vi "doComms.vi"(1 "Initialization":T1={"connID"=refnum, "client"="", "OpenFP"=TRUE, "useAuthentication"=FALSE, "DSN"="", "Package Size"=1, "Sending Rate (ms)"=100, "error"={"status"=FALSE, "code"=0, "source"=""}} {"Sending Rate (ms)" min=1 max=1000 step=1; "Package Size" min=1 max=1000 step=1}) -> ()   [LabVIEW 2010]
panel:
  out "starttime":string
  out "endtime":string
  out "Indicators formated":cluster{"name":string, "type desc":i16[]}[](array[cluster])
  out "Controls formated":cluster{"name":string, "type desc":i16[]}[](array[cluster])
  out "output Indicators":cluster{"name":string, "type desc":i16[]}[](array[cluster])
  out "output Controls":cluster{"name":string, "type desc":i16[]}[](array[cluster])
  out "vi reference":refnum<vi>
  out "Execution: State VI":T2(ring)
  out "Application":string
  out "Application absolute path":path
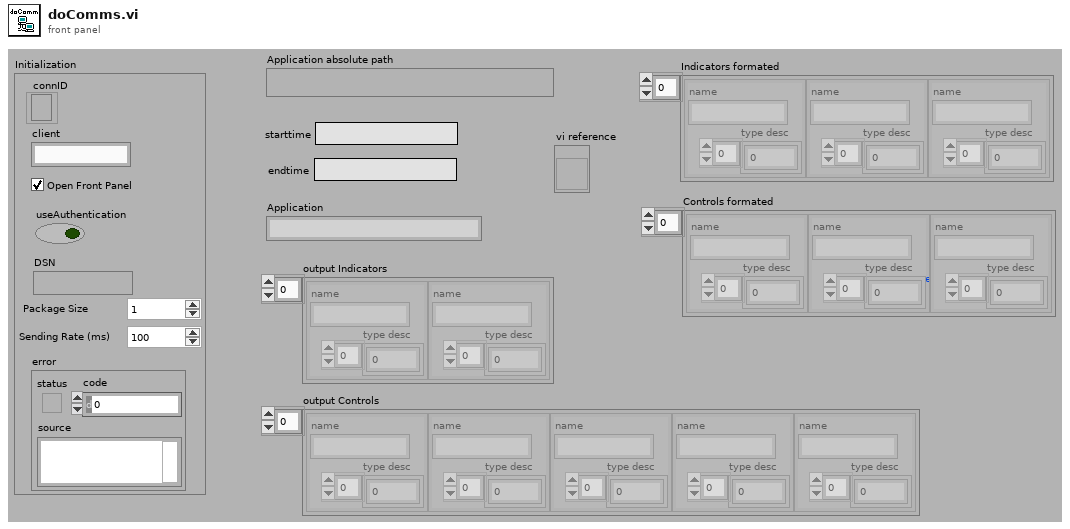
[diagram p1: front panel]
types:
  T1 = cluster{"connID":refnum<k5>, "client":string, "OpenFP":bool, "useAuthentication":bool, "DSN":string, "Package Size":u32, "Sending Rate (ms)":u32, "error":errorcluster}
  T2 = enum16{"Bad", "Idle", "Run top level", "Running"}
  T3 = enum32{"Bad", "Idle", "Run top level", "Running"}
  T4 = enum16{"open", "replace", "create", "open or create", "replace or create", "replace or create with confirmation"}
  T5 = typedef "imagedata.ctl" = cluster{"image type":i32, "image depth":i32, "image":u8[], "mask":u8[], "colors":u32[], "Rectangle":cluster{"left":i16, "top":i16, "right":i16, "bottom":i16}}
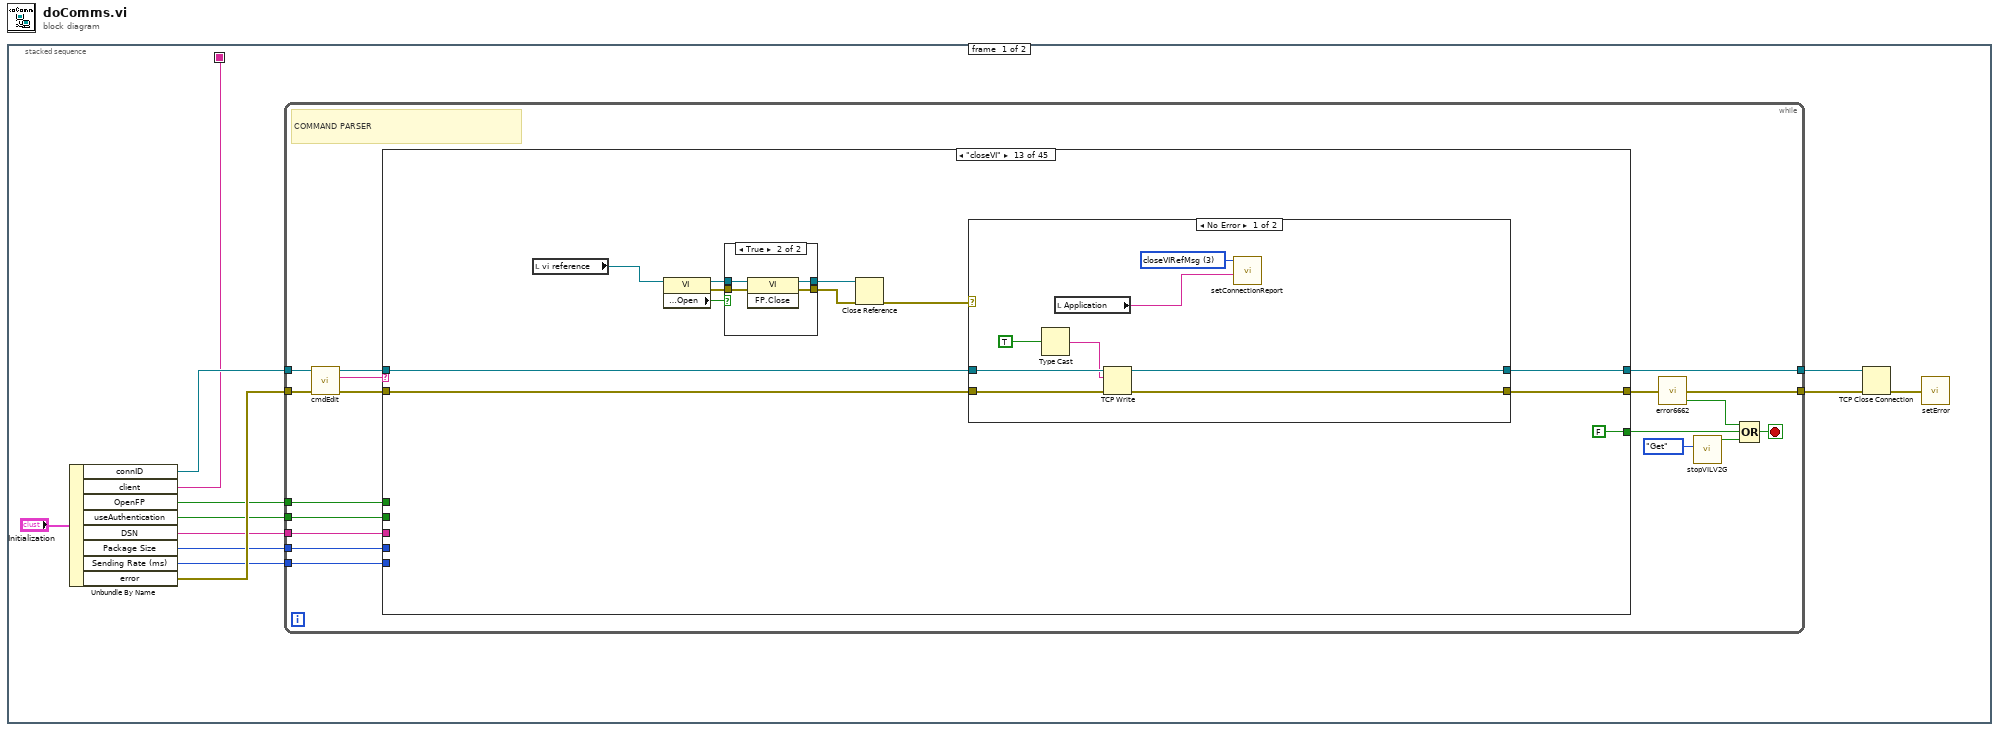
[diagram p0: block diagram]
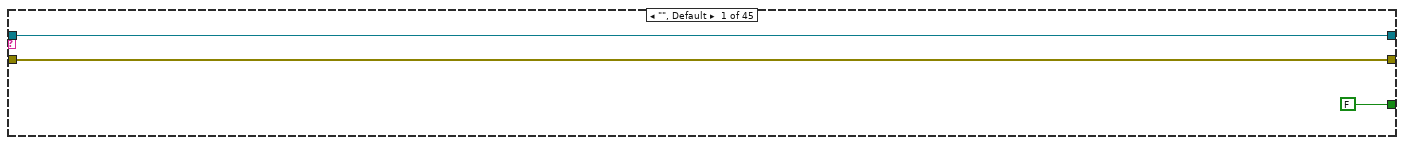
[diagram p2: hidden frame]
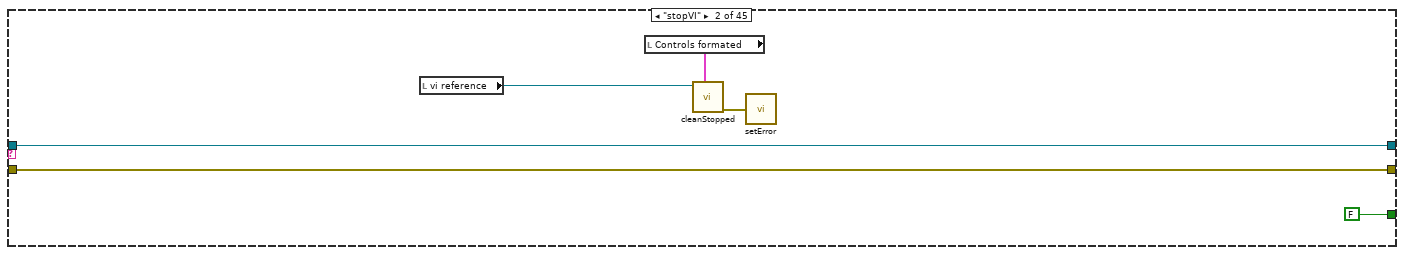
[diagram p3: hidden frame]
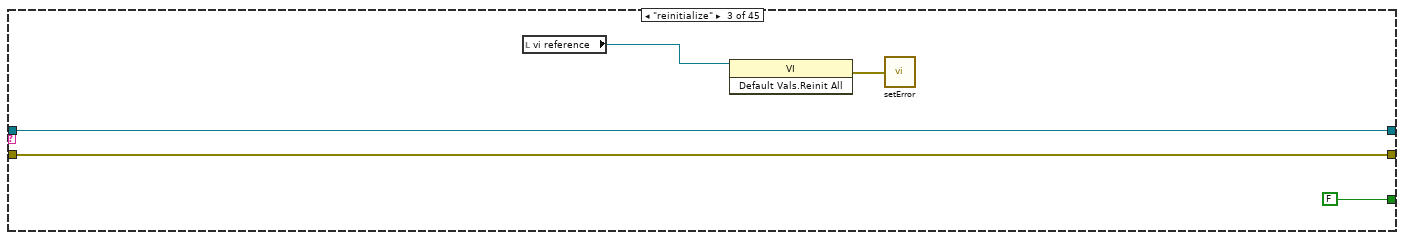
[diagram p4: hidden frame]
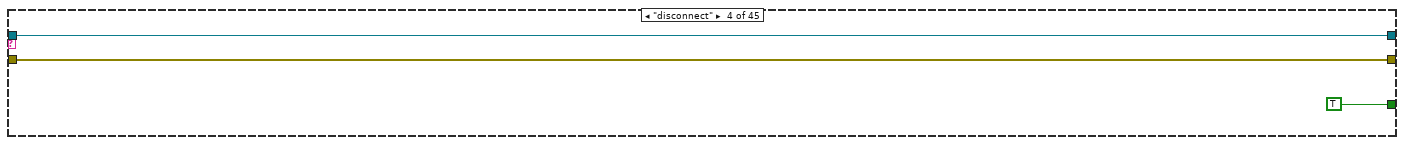
[diagram p5: hidden frame]
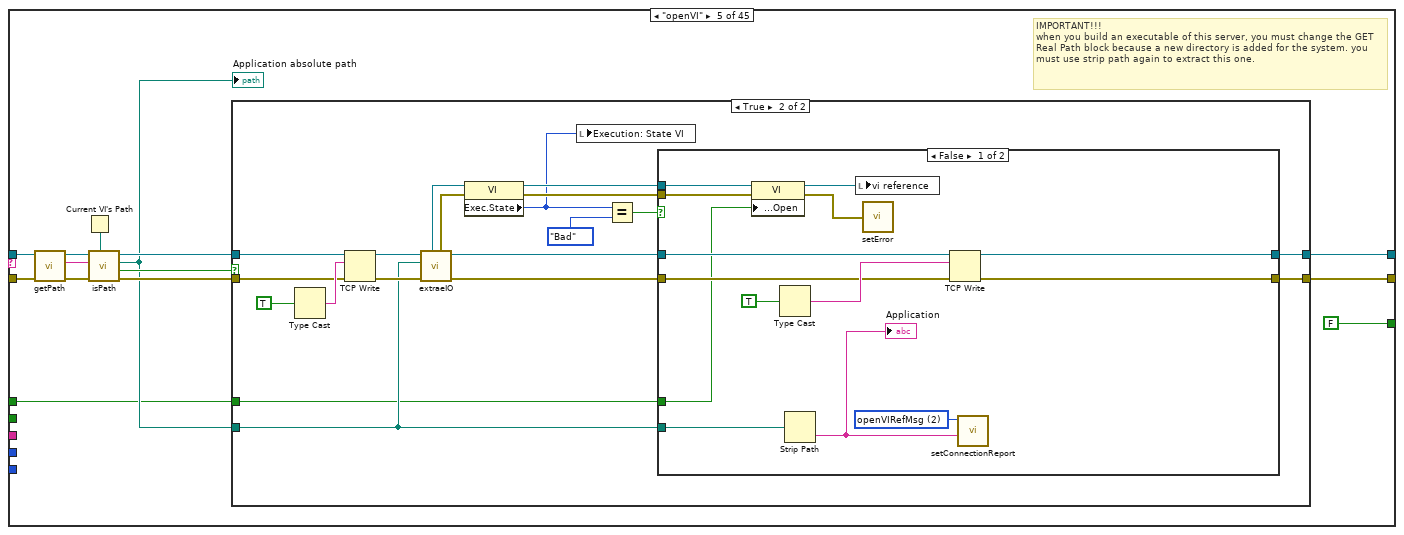
[diagram p6: hidden frame]
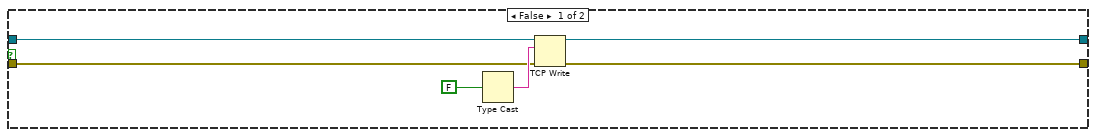
[diagram p7: hidden frame]
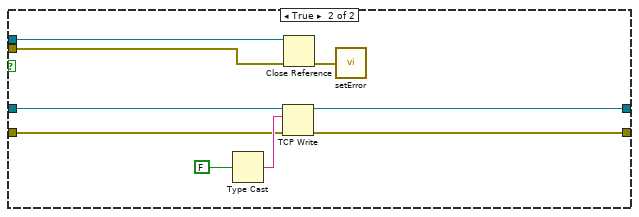
[diagram p8: hidden frame]
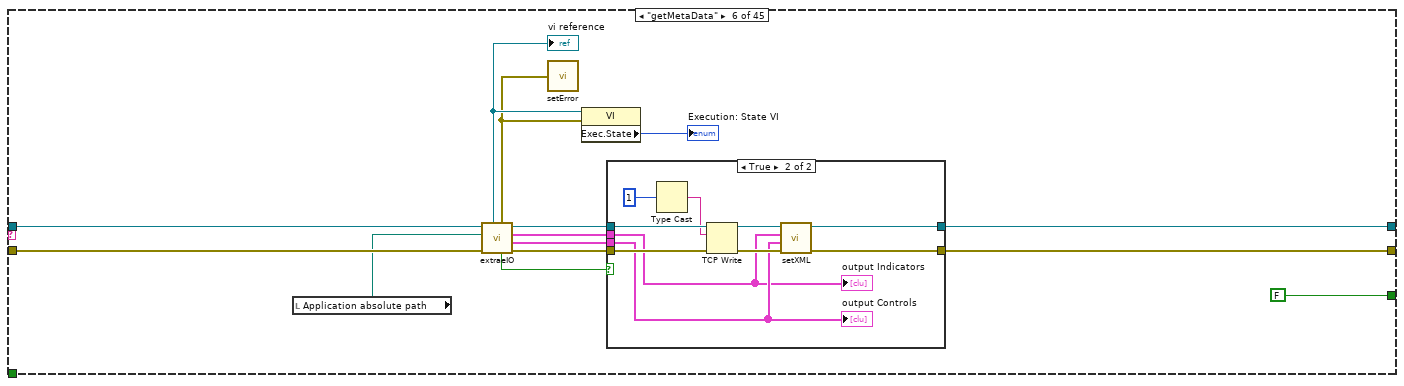
[diagram p9: hidden frame]
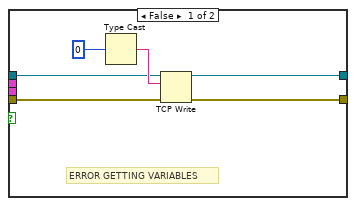
[diagram p10: hidden frame]
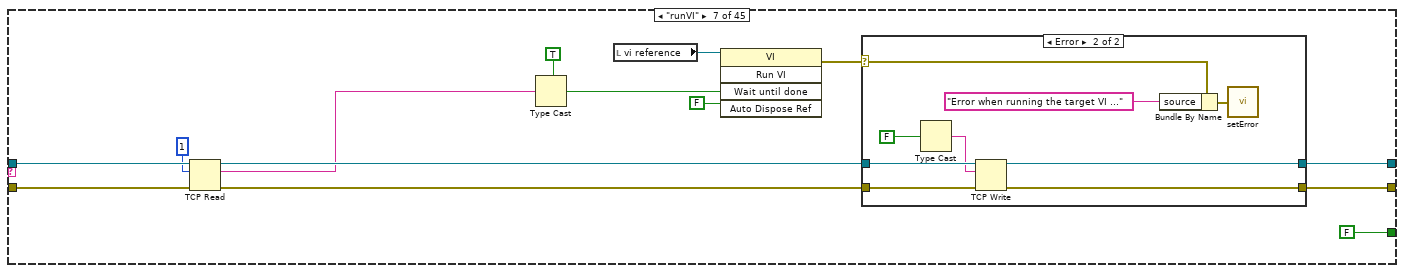
[diagram p11: hidden frame]
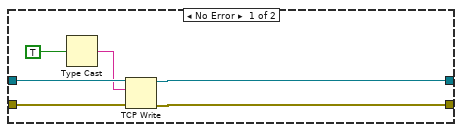
[diagram p12: hidden frame]
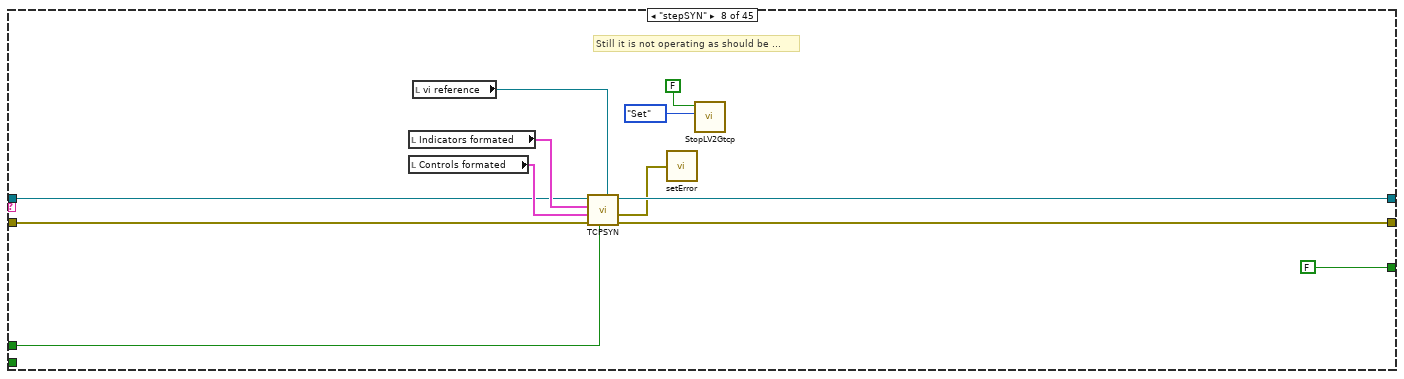
[diagram p13: hidden frame]
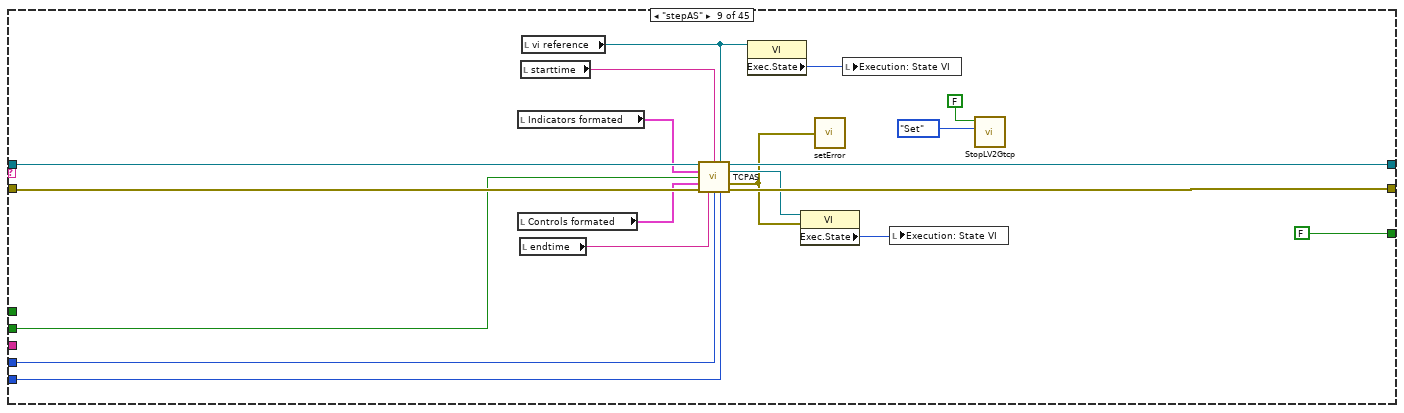
[diagram p14: hidden frame]
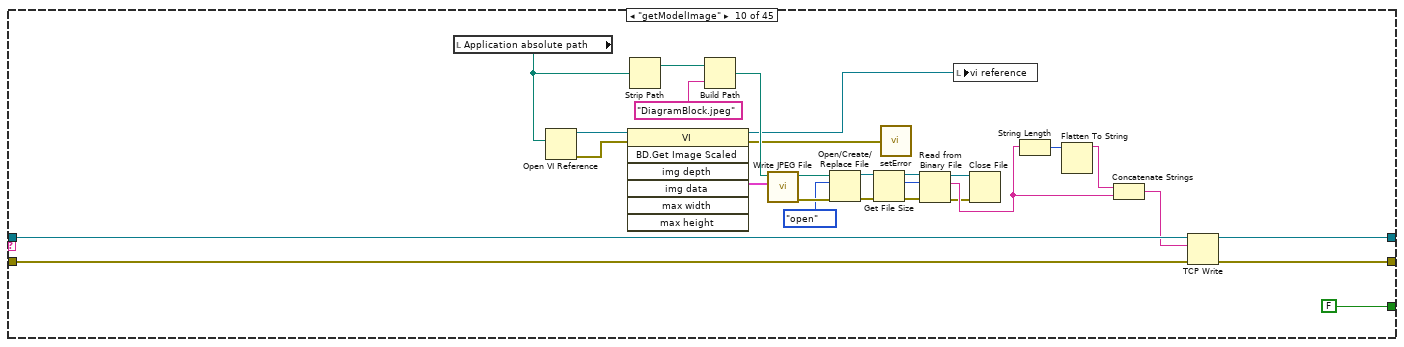
[diagram p15: hidden frame]
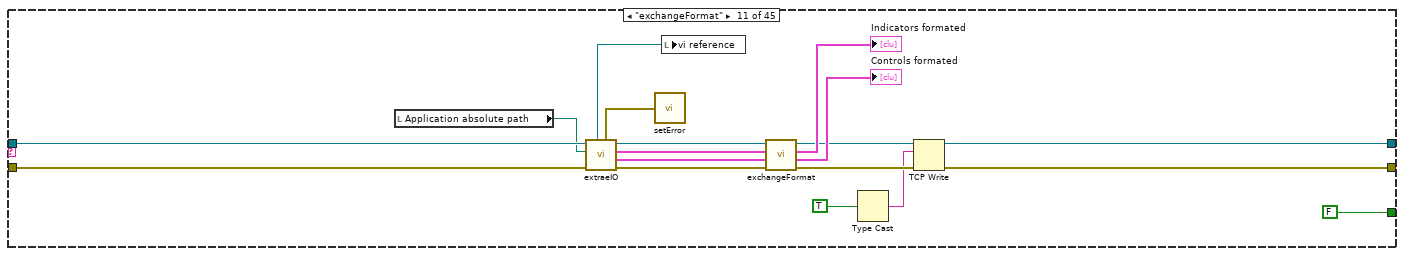
[diagram p16: hidden frame]
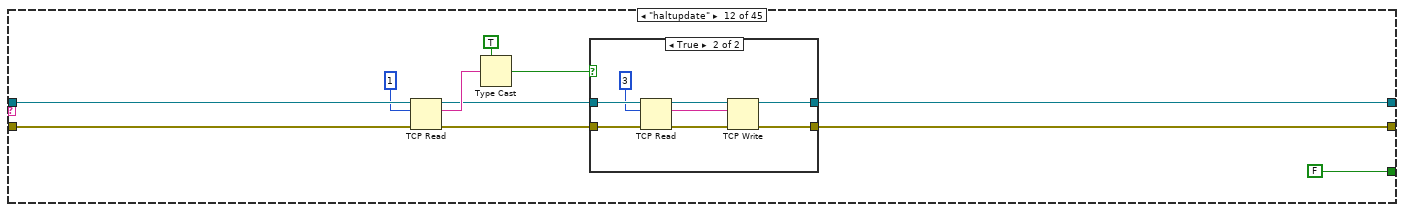
[diagram p17: hidden frame]
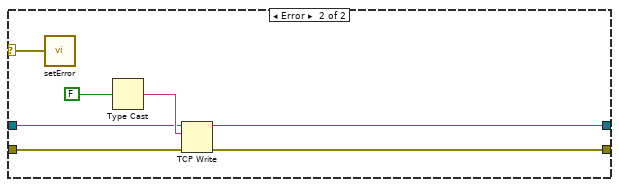
[diagram p19: hidden frame]
diagram:
  n1 = stacked-sequence {
    seq-local: [w1 _] -> [_ w1190]
    frame #0 {
      n2 = Unbundle By Name("Initialization") -> ("connID"=w8:refnum<k5>, "client"=w1:string, "OpenFP"=w5:bool, "useAuthentication"=w6:bool, "DSN"=w2:string, "Package Size"=w4:u32, "Sending Rate (ms)"=w3:u32, "error"=w7:errorcluster)
      n3 = while {
        tunnel: w8 -> [w29]
        tunnel: w7 -> [w28]
        tunnel: [w23] -> w12
        tunnel: [w30] -> w11
        tunnel: w6 -> [w17]
        tunnel: w5 -> [w16]
        tunnel: w4 -> [w15]
        tunnel: w3 -> [w14]
        tunnel: w2 -> [w13]
        stop <- w22 stop-if-true
        # "COMMAND PARSER"
        n4 = call "cmdEdit.vi"("error in (no error)"=w28, "connection ID"=w29) -> ("error out"=w26:errorcluster, "Command"=w25:string, "connection ID out"=w27:refnum<k5>)  [unwired: 7 out]
        n5 = case shown="\"closeVI\"" w25 {
          tunnel: w27 -> [w33 w38 w43 w47 w57 w117 w152 w177 w196 w221 w245 w256 w271 w314 w351 w359 w384 w407 w430 w461 w485 w515 w551 w590 w623 w661 w700 w739 w780 w827 w871 w890 w912 w934 w955 w978 w1000 w1022 w1044 w1065 w1088 w1110 w1132 w1150 w1173]
          tunnel: w26 -> [w32 w37 w42 w46 w56 w116 w151 w176 w195 w220 w244 w255 w270 w313 w350 w358 w383 w406 w429 w460 w484 w516 w550 w589 w622 w660 w699 w738 w779 w826 w870 w889 w911 w933 w954 w977 w999 w1021 w1043 w1064 w1087 w1109 w1131 w1149 w1172]
          tunnel: [w32 w37 w42 w46 w51 w122 w148 w175 w192 w225 w232 w246 w267 w303 w350 w357 w382 w404 w428 w459 w483 w517 w549 w581 w625 w658 w697 w737 w773 w825 w865 w888 w910 w932 w953 w976 w998 w1020 w1042 w1062 w1085 w1108 w1130 w1152 w1171] -> w24
          tunnel: [w33 w38 w43 w47 w52 w123 w149 w174 w191 w226 w231 w247 w268 w304 w351 w356 w381 w405 w427 w458 w482 w518 w552 w582 w624 w659 w698 w736 w774 w824 w863 w887 w909 w931 w952 w975 w997 w1019 w1041 w1063 w1086 w1107 w1129 w1153 w1170] -> w30
          tunnel: [FALSE FALSE FALSE TRUE FALSE FALSE FALSE FALSE FALSE FALSE FALSE FALSE FALSE FALSE FALSE FALSE FALSE FALSE FALSE FALSE FALSE FALSE FALSE FALSE FALSE FALSE FALSE FALSE FALSE FALSE FALSE FALSE FALSE FALSE FALSE FALSE FALSE FALSE FALSE FALSE FALSE FALSE FALSE FALSE FALSE] -> w20
          tunnel: w17 -> [_ _ _ _ _ _ _ _ w188 _ _ _ _ _ _ _ _ _ _ _ _ _ _ _ _ _ _ _ _ _ _ _ _ _ _ _ _ _ _ _ _ _ _ _ _]
          tunnel: w16 -> [_ _ _ _ w48 _ _ w169 _ _ _ _ _ _ _ _ _ _ _ _ _ _ _ _ _ _ _ _ _ _ _ _ _ _ _ _ _ _ _ _ _ _ _ _ _]
          tunnel: w15 -> [_ _ _ _ _ _ _ _ w182 _ _ _ _ _ _ _ _ _ _ _ _ _ _ _ _ _ _ _ _ _ _ _ _ _ _ _ _ _ _ _ _ _ _ _ _]
          tunnel: w14 -> [_ _ _ _ _ _ _ _ w181 _ _ _ _ _ _ _ _ _ _ _ _ _ _ _ _ _ _ _ _ _ _ _ _ _ _ _ _ _ _ _ _ _ _ _ _]
          tunnel: w13 -> [_ _ _ _ _ _ _ _ _ _ _ _ _ w300 _ _ _ _ _ _ _ _ _ _ _ _ _ _ _ _ _ _ _ _ _ _ _ _ _ _ _ _ _ _ _]
          frame "", Default {
          }
          frame "stopVI" {
            n6 = local read "vi reference"() -> (w36:refnum<vi>)
            n7 = local read "Controls formated"() -> (w35:cluster{"name":string, "type desc":i16[]}[])
            n8 = call "cleanStopped.vi"("input Controls"=w35, "vi reference in"=w36) -> ("error out"=w34:errorcluster)  [unwired: 1 in, 8 out]
            n9 = call "setError.vi"("error"=w34) -> ()  [unwired: 1 out]
          }
          frame "reinitialize" {
            n10 = local read "vi reference"() -> (w41:refnum<vi>)
            n11 = invoke class="VI" method="Default Vals.Reinit All"(reference=w41) -> (error out=w40:errorcluster)  [unwired: 2 in, 2 out]
            n12 = call "setError.vi"("error"=w40) -> ()  [unwired: 1 out]
          }
          frame "disconnect" {
          }
          frame "openVI" {
            # "IMPORTANT!!!\nwhen you build an executable of this server, you must change the GET Real Path block because a new directory is added for the system. you must use strip path again to extract this one."
            n13 = call "getPath.vi"("error in TCP"=w56, "connection ID in"=w57) -> ("error out TCP"=w58:errorcluster, "name vi"=w61:string, "connection ID out"=w59:refnum<k5>)  [unwired: 7 out]
            n14 = Current VI's Path() -> (path=w60:path)
            n15 = call "isPath.vi"("path Current VI"=w60, "error in TCP"=w58, "string Path in"=w61, "connection ID in"=w59) -> ("error out TCP"=w54:errorcluster, "Path is Ok?"=w55:bool, "absolute path"=w49:path, "connection ID out"=w53:refnum<k5>)  [unwired: 4 out]
            "Application absolute path" <- w49
            n16 = case shown="True" w55 {
              tunnel: w54 -> [w64 w83]
              tunnel: w53 -> [w65 w84]
              tunnel: [w62 w71] -> w52
              tunnel: [w63 w72] -> w51
              tunnel: w49 -> [_ w70]
              tunnel: w48 -> [_ w68]
              frame False {
                n17 = Type Cast(x=FALSE) -> (*(type *) &x=w67:string)  [unwired: 1 out]
                n18 = TCP Write(connection ID=w65, data in=w67, error in (no error)=w64) -> (connection ID out=w62:refnum<k5>, error out=w63:errorcluster)  [unwired: 2 out]
              }
              frame True {
                n19 = Type Cast(x=TRUE) -> (*(type *) &x=w86:string)  [unwired: 1 out]
                n20 = TCP Write(connection ID=w84, data in=w86, error in (no error)=w83) -> (connection ID out=w82:refnum<k5>, error out=w81:errorcluster)  [unwired: 2 out]
                n21 = call "extraeIO.vi"("error in TCP"=w81, "path"=w70, "connection IDin"=w82) -> ("error out TCP"=w73:errorcluster, "connection ID out"=w74:refnum<k5>, "error out"=w79:errorcluster, "vi reference"=w80:refnum<vi>)  [unwired: 5 out]
                n22 = property class="VI"(reference=w80, error in=w79) -> (reference out=w76:refnum<vi>, error out=w75:errorcluster, "Exec.State"=w69:T3)
                n23 = local write "Execution: State VI"(w69) -> ()
                n24 = Equal?(x=w69, y=T3."Bad") -> (x = y?=w78:bool)
                n25 = case shown="False" w78 {
                  tunnel: w76 -> [w92 w106]
                  tunnel: w75 -> [w91 w107]
                  tunnel: w74 -> [w96 w105]
                  tunnel: w73 -> [w95 w104]
                  tunnel: [w94 w103] -> w72
                  tunnel: [w93 w102] -> w71
                  tunnel: w70 -> [w97 _]
                  tunnel: w68 -> [w87 _]
                  frame False {
                    w88 = u16 2 items=["connectedMsg", "disconnectedMsg", "openVIRefMsg", "closeVIRefMsg"] ("Type of Message")
                    n26 = property class="VI"(reference=w92, error in=w91, "Front Panel.Open"=w87) -> (reference out=w98:refnum<vi>, error out=w90:errorcluster)
                    n27 = Type Cast(x=TRUE) -> (*(type *) &x=w100:string)  [unwired: 1 out]
                    n28 = Strip Path(path=w97) -> (name=w89:string)  [unwired: 1 out]
                    "Application" <- w89
                    n29 = local write "vi reference"(w98) -> ()
                    n30 = call "setError.vi"("error"=w90) -> ()  [unwired: 1 out]
                    n31 = TCP Write(connection ID=w96, data in=w100, error in (no error)=w95) -> (connection ID out=w93:refnum<k5>, error out=w94:errorcluster)  [unwired: 2 out]
                    n32 = call "setConnectionReport.vi"("string"=w89, "Type of Message"=w88) -> ()  [unwired: 10 in]
                  }
                  frame True {
                    n33 = Type Cast(x=FALSE) -> (*(type *) &x=w109:string)  [unwired: 1 out]
                    n34 = TCP Write(connection ID=w105, data in=w109, error in (no error)=w104) -> (connection ID out=w102:refnum<k5>, error out=w103:errorcluster)  [unwired: 2 out]
                    n35 = Close Reference(reference=w106, error in (no error)=w107) -> (error out=w101:errorcluster)
                    n36 = call "setError.vi"("error"=w101) -> ()  [unwired: 1 out]
                  }
                }
              }
            }
          }
          frame "getMetaData" {
            n37 = local read "Application absolute path"() -> (w115:path)
            n38 = call "extraeIO.vi"("error in TCP"=w116, "path"=w115, "connection IDin"=w117) -> ("error out TCP"=w119:errorcluster, "output Controls"=w113:cluster{"name":string, "type desc":i16[]}[], "output Indicators"=w120:cluster{"name":string, "type desc":i16[]}[], "connection ID out"=w118:refnum<k5>, "it is ok?"=w114:bool, "error out"=w110:errorcluster, "vi reference"=w112:refnum<vi>)  [unwired: 2 out]
            "vi reference" <- w112
            n39 = call "setError.vi"("error"=w110) -> ()  [unwired: 1 out]
            n40 = property class="VI"(reference=w112, error in=w110) -> ("Exec.State"=→"Execution: State VI":T3)  [unwired: 2 out]
            n41 = case shown="True" w114 {
              tunnel: w119 -> [w129 w136]
              tunnel: w120 -> [_ w130]
              tunnel: w113 -> [_ w131]
              tunnel: [w127 w139] -> w123
              tunnel: [w128 w138] -> w122
              tunnel: w118 -> [w124 w137]
              frame False {
                # "ERROR GETTING VARIABLES"
                n42 = Type Cast(x=0) -> (*(type *) &x=w126:string)  [unwired: 1 out]
                n43 = TCP Write(connection ID=w124, data in=w126, error in (no error)=w129) -> (connection ID out=w127:refnum<k5>, error out=w128:errorcluster)  [unwired: 2 out]
              }
              frame True {
                n44 = Type Cast(x=1) -> (*(type *) &x=w132:string)  [unwired: 1 out]
                n45 = TCP Write(connection ID=w137, data in=w132, error in (no error)=w136) -> (connection ID out=w134:refnum<k5>, error out=w135:errorcluster)  [unwired: 2 out]
                n46 = call "setXML.vi"("error in"=w135, "Controls filtered"=w131, "Indicators filtered"=w130, "connection ID in"=w134) -> ("error out"=w138:errorcluster, "connection ID out"=w139:refnum<k5>)  [unwired: 6 out]
                "output Indicators" <- w130
                "output Controls" <- w131
              }
            }
          }
          frame "runVI" {
            n47 = TCP Read(connection ID=w152, bytes to read=1, error in (no error)=w151) -> (connection ID out=w147:refnum<k5>, data out=w142:string, error out=w146:errorcluster)  [unwired: 2 out]
            n48 = Type Cast(type=TRUE, x=w142) -> (*(type *) &x=w145:bool)
            n49 = local read "vi reference"() -> (w141:refnum<vi>)
            n50 = invoke class="VI" method="Run VI"(reference=w141, "Wait until done"=w145, "Auto Dispose Ref"=FALSE ("Auto Dispose Reference")) -> (error out=w150:errorcluster)  [unwired: 2 in, 4 out]
            n51 = case shown="Error" w150 {
              selector: w150 -> [_ w161]
              tunnel: w147 -> [w159 w168]
              tunnel: w146 -> [w158 w167]
              tunnel: [w157 w166] -> w149
              tunnel: [w156 w165] -> w148
              frame No Error {
                n52 = Type Cast(x=TRUE) -> (*(type *) &x=w154:string)  [unwired: 1 out]
                n53 = TCP Write(connection ID=w159, data in=w154, error in (no error)=w158) -> (connection ID out=w157:refnum<k5>, error out=w156:errorcluster)  [unwired: 2 out]
              }
              frame Error {
                n54 = Type Cast(x=FALSE) -> (*(type *) &x=w163:string)  [unwired: 1 out]
                n55 = TCP Write(connection ID=w168, data in=w163, error in (no error)=w167) -> (connection ID out=w166:refnum<k5>, error out=w165:errorcluster)  [unwired: 2 out]
                n56 = Bundle By Name(cluster=w161, "source"="Error when running the target VI ...") -> (w160:errorcluster)
                n57 = call "setError.vi"("error"=w160) -> ()  [unwired: 1 out]
              }
            }
          }
          frame "stepSYN" {
            # "Still it is not operating as should be ..."
            n58 = local read "Indicators formated"() -> (w180:cluster{"name":string, "type desc":i16[]}[])
            n59 = local read "Controls formated"() -> (w179:cluster{"name":string, "type desc":i16[]}[])
            n60 = local read "vi reference"() -> (w178:refnum<vi>)
            n61 = call "TCPSYN.vi"("vi reference"=w178, "Front Panel Window:Open"=w169, "error in TCP"=w176, "input Controls"=w179, "input Indicators"=w180, "connection ID in"=w177) -> ("error TCP out"=w175:errorcluster, "error out"=w170:errorcluster, "connection ID out"=w174:refnum<k5>)  [unwired: 1 in, 2 out]
            n62 = call "setError.vi"("error"=w170) -> ()  [unwired: 1 out]
            n63 = call "StopLV2Gtcp.vi"("Mode"=enum16{"Init", "Get", "Set"}."Set", "Stop IN"=FALSE) -> ()  [unwired: 10 out]
          }
          frame "stepAS" {
            n64 = local read "Indicators formated"() -> (w194:cluster{"name":string, "type desc":i16[]}[])
            n65 = local read "Controls formated"() -> (w193:cluster{"name":string, "type desc":i16[]}[])
            n66 = local read "endtime"() -> (w189:string)
            n67 = local read "starttime"() -> (w190:string)
            n68 = local read "vi reference"() -> (w187:refnum<vi>)
            n69 = call "TCPAS.vi"("connection ID in"=w196, "starttime"=w190, "vi reference"=w187, "input Indicators"=w194, "rejectbyendtime"=w188, "input Controls"=w193, "error in TCP"=w195, "endtime"=w189, "packageSize"=w182, "Sent rate (ms)"=w181) -> ("connection ID out"=w191:refnum<k5>, "vi reference"=w185:refnum<vi>, "error out"=w183:errorcluster, "error TCP out"=w192:errorcluster)  [unwired: 1 in, 1 out]
            n70 = property class="VI"(reference=w187) -> ("Exec.State"=w186:T3)  [unwired: 1 in, 2 out]
            n71 = property class="VI"(reference=w185, error in=w183) -> ("Exec.State"=w184:T3)  [unwired: 2 out]
            n72 = call "setError.vi"("error"=w183) -> ()  [unwired: 1 out]
            n73 = local write "Execution: State VI"(w186) -> ()
            n74 = local write "Execution: State VI"(w184) -> ()
            n75 = call "StopLV2Gtcp.vi"("Mode"=enum16{"Init", "Get", "Set"}."Set", "Stop IN"=FALSE) -> ()  [unwired: 10 out]
          }
          frame "getModelImage" {
            n76 = local read "Application absolute path"() -> (w219:path)
            n77 = Open VI Reference(vi path=w219) -> (vi reference=w218:refnum<vi>, error out=w217:errorcluster)  [unwired: 1 in, 4 out]
            n78 = invoke class="VI" method="BD.Get Image Scaled"(reference=w218, error in=w217) -> (reference out=w216:refnum<vi>, error out=w200:errorcluster, "img data"=w215:T5)  [unwired: 5 in, 4 out]
            n79 = Strip Path(path=w219) -> (stripped path=w224:path)  [unwired: 1 out]
            n80 = Build Path(base path=w224, name or relative path="DiagramBlock.jpeg") -> (appended path=w222:path)
            n81 = call <vilib>:"Write JPEG File.vi"("image data"=w215, "path to JPEG file"=w222) -> ("error out"=w208:errorcluster, "path"=w209:path)  [unwired: 1 in, 7 out]
            n82 = Open/Create/Replace File(file path (use dialog)=w209, error in=w208, operation (0:open)=T4."open") -> (refnum out=w210:refnum<file>, error out=w211:errorcluster)  [unwired: 4 out]
            n83 = Get File Size(file=w210, error in=w211) -> (refnum out=w206:refnum<file>, size (in bytes)=w205:i64, 0:w204:errorcluster)
            n84 = call "setError.vi"("error"=w200) -> ()  [unwired: 1 out]
            n85 = Read from Binary File(8:w204, 10:w205, 11:w206) -> (0:w202:errorcluster, 2:w214:string, 3:w203:refnum<file>)  [unwired: 4 out]
            n86 = local write "vi reference"(w216) -> ()
            n87 = Close File(refnum=w203, error in=w202) -> ()  [unwired: 2 out]
            n88 = String Length(string=w214) -> (length=w201:i32)
            n89 = Flatten To String(anything=w201) -> (data string=w213:string)  [unwired: 1 in, 4 out]
            n90 = Concatenate Strings(w213, w214) -> (w212:string)
            n91 = TCP Write(connection ID=w221, data in=w212, error in (no error)=w220) -> (connection ID out=w226:refnum<k5>, error out=w225:errorcluster)  [unwired: 2 out]
          }
          frame "exchangeFormat" {
            n92 = local read "Application absolute path"() -> (w243:path)
            n93 = call "extraeIO.vi"("error in TCP"=w244, "path"=w243, "connection IDin"=w245) -> ("error out TCP"=w239:errorcluster, "output Controls"=w237:cluster{"name":string, "type desc":i16[]}[], "output Indicators"=w238:cluster{"name":string, "type desc":i16[]}[], "connection ID out"=w240:refnum<k5>, "error out"=w228:errorcluster, "vi reference"=w241:refnum<vi>)  [unwired: 3 out]
            n94 = call "setError.vi"("error"=w228) -> ()  [unwired: 1 out]
            n95 = local write "vi reference"(w241) -> ()
            n96 = call "exchangeFormat.vi"("error in TCP"=w239, "input Controls"=w237, "input Indicators"=w238, "connection ID in"=w240) -> ("error out TCP"=w233:errorcluster, "output Controls"=→"Controls formated":cluster{"name":string, "type desc":i16[]}[], "output Indicators"=→"Indicators formated":cluster{"name":string, "type desc":i16[]}[], "connection ID out"=w234:refnum<k5>)  [unwired: 4 out]
            n97 = Type Cast(x=TRUE) -> (*(type *) &x=w230:string)  [unwired: 1 out]
            n98 = TCP Write(connection ID=w234, data in=w230, error in (no error)=w233) -> (connection ID out=w231:refnum<k5>, error out=w232:errorcluster)  [unwired: 2 out]
          }
          frame "haltupdate" {
            n99 = TCP Read(connection ID=w256, bytes to read=1, error in (no error)=w255) -> (connection ID out=w249:refnum<k5>, data out=w253:string, error out=w248:errorcluster)  [unwired: 2 out]
            n100 = Type Cast(type=TRUE, x=w253) -> (*(type *) &x=w251:bool)
            n101 = case shown="True" w251 {
              tunnel: w249 -> [w258 w266]
              tunnel: w248 -> [w257 w265]
              tunnel: [w258 w260] -> w247
              tunnel: [w257 w259] -> w246
              frame False {
              }
              frame True {
                n102 = TCP Read(connection ID=w266, bytes to read=3, error in (no error)=w265) -> (connection ID out=w264:refnum<k5>, data out=w262:string, error out=w263:errorcluster)  [unwired: 2 out]
                n103 = TCP Write(connection ID=w264, data in=w262, error in (no error)=w263) -> (connection ID out=w260:refnum<k5>, error out=w259:errorcluster)  [unwired: 2 out]
              }
            }
          }
          frame "closeVI" {
            n104 = local read "vi reference"() -> (w273:refnum<vi>)
            n105 = property class="VI"(reference=w273) -> (reference out=w276:refnum<vi>, error out=w277:errorcluster, "Front Panel.Open"=w278:bool)  [unwired: 1 in]
            n106 = case shown="True" w278 {
              tunnel: w276 -> [w295 w299]
              tunnel: w277 -> [w294 w296]
              tunnel: [w295 w298] -> w274
              tunnel: [w294 w297] -> w275
              frame False {
              }
              frame True {
                n107 = invoke class="VI" method="FP.Close"(reference=w299, error in=w296) -> (reference out=w298:refnum<vi>, error out=w297:errorcluster)  [unwired: 1 in, 1 out]
              }
            }
            n108 = Close Reference(reference=w274, error in (no error)=w275) -> (error out=w272:errorcluster)
            n109 = case shown="No Error" w272 {
              selector: w272 -> [_ w287]
              tunnel: w271 -> [w285 w291]
              tunnel: w270 -> [w286 w290]
              tunnel: [w282 w289] -> w268
              tunnel: [w281 w288] -> w267
              frame No Error {
                w280 = u16 3 items=["connectedMsg", "disconnectedMsg", "openVIRefMsg", "closeVIRefMsg"] ("Type of Message")
                n110 = Type Cast(x=TRUE) -> (*(type *) &x=w283:string)  [unwired: 1 out]
                n111 = local read "Application"() -> (w279:string)
                n112 = TCP Write(connection ID=w285, data in=w283, error in (no error)=w286) -> (connection ID out=w282:refnum<k5>, error out=w281:errorcluster)  [unwired: 2 out]
                n113 = call "setConnectionReport.vi"("string"=w279, "Type of Message"=w280) -> ()  [unwired: 10 in]
              }
              frame Error {
                n114 = call "setError.vi"("error"=w287) -> ()  [unwired: 1 out]
                n115 = Type Cast(x=FALSE) -> (*(type *) &x=w292:string)  [unwired: 1 out]
                n116 = TCP Write(connection ID=w291, data in=w292, error in (no error)=w290) -> (connection ID out=w289:refnum<k5>, error out=w288:errorcluster)  [unwired: 2 out]
              }
            }
          }
          frame "authenticate" {
            # "TCP reference ->"
            # "TCP reference ->"
            # "Execution flow:\n1. Receiving user's credentials.\n2. Checking user's credentials with database.\n3. Checking whether timeslot is correct.\n4. Sending authentication result to client."
            # "2."
            # "1."
            # "4."
            n117 = call "userpassReceptor.vi"("error in (no error)"=w313, "connection ID"=w314) -> ("error out"=w311:errorcluster, "password"=w309:string, "user"=w310:string, "connection ID out"=w312:refnum<k5>)  [unwired: 2 out]
            n118 = call "CheckUserPass.vi"("ConnectionString"=w300, "error in"=w311, "password"=w309, "user"=w310, "connection ID in"=w312) -> ("error out"=w316:errorcluster, "endtime"=w318:string, "starttime"=w319:string, "connection ID out"=w315:refnum<k5>, "result"=w317:bool)  [unwired: 2 out]
            n119 = case shown="True" w317 {
              tunnel: w319 -> [w324 w335]
              tunnel: w318 -> [w323 w334]
              tunnel: [w324 w337] -> w302
              tunnel: [w323 w336] -> w301
              tunnel: [w322 w338] -> w305
              tunnel: w316 -> [w320 w330]
              tunnel: w315 -> [w321 w329]
              tunnel: [w321 w326] -> w307
              tunnel: [w320 w325] -> w306
              frame False {
                w322 = 0 items=["user and pass no exist", "no match with timeslot", "user ok"] ("result")
              }
              frame True {
                # "3."
                n120 = call "CheckTimeSlot.vi"("connection ID in"=w329, "starttime"=w335, "endtime"=w334, "error in"=w330) -> ("Timeslot In Range?"=w331:bool, "connection ID out"=w328:refnum<k5>, "starttime out"=w333:string, "endtime out"=w332:string, "error out"=w327:errorcluster)
                n121 = case shown="True" w331 {
                  tunnel: w333 -> [w342 w347]
                  tunnel: w332 -> [w341 w346]
                  tunnel: [w343 w348] -> w338
                  tunnel: [w342 w347] -> w337
                  tunnel: [w341 w346] -> w336
                  tunnel: w328 -> [w340 w345]
                  tunnel: w327 -> [w339 w344]
                  tunnel: [w340 w345] -> w326
                  tunnel: [w339 w344] -> w325
                  frame False {
                    w343 = 1 items=["user and pass no exist", "no match with timeslot", "user ok"] ("result")
                  }
                  frame True {
                    w348 = 2 items=["user and pass no exist", "no match with timeslot", "user ok"] ("result")
                  }
                }
              }
            }
            "starttime" <- w302
            "endtime" <- w301
            n122 = call "SendResult.vi"("result"=w305, "error in (no error)"=w306, "endtime in"=w301, "starttime in"=w302, "connection ID in"=w307) -> ("error out"=w303:errorcluster, "connection ID out"=w304:refnum<k5>)  [unwired: 5 out]
          }
          frame "clientKeepAlive" {
          }
          frame "setBoolean" {
            n123 = TCP Read(connection ID=w359, bytes to read=4, error in (no error)=w358) -> (connection ID out=w368:refnum<k5>, data out=w371:string, error out=w367:errorcluster)  [unwired: 2 out]
            n124 = Type Cast(type=0, x=w371) -> (*(type *) &x=w369:i32)
            n125 = TCP Read(connection ID=w368, bytes to read=w369, error in (no error)=w367) -> (connection ID out=w365:refnum<k5>, data out=w362:string, error out=w366:errorcluster)  [unwired: 2 out]
            n126 = TCP Read(connection ID=w365, bytes to read=1, error in (no error)=w366) -> (connection ID out=w356:refnum<k5>, data out=w363:string, error out=w357:errorcluster)  [unwired: 2 out]
            n127 = call "deleteEndString.vi"("chars to delete"=5, "string in"=w362) -> ("substring out"=w361:string)  [unwired: 9 out]
            n128 = local read "Controls formated"() -> (w353:cluster{"name":string, "type desc":i16[]}[])
            n129 = local read "vi reference"() -> (w354:refnum<vi>)
            n130 = call "searchElement.vi"("input"=w353, "name"=w361) -> ("output"=w374:cluster{"name":string, "type desc":i16[]})  [unwired: 9 out]
            n131 = Unbundle By Name(w374) -> ("name"=w373:string, "type desc"=w372:i16[])
            n132 = invoke class="VI" method="Ctrl Val.Set (Deprecated)"(reference=w354, "Control Name"=w373, "Type Descriptor"=w372, "Flattened Data"=w363) -> (error out=w352:errorcluster)  [unwired: 2 in, 5 out]
            n133 = call "setError.vi"("error"=w352) -> ()  [unwired: 1 out]
          }
          frame "setInt" {
            n134 = TCP Read(connection ID=w384, bytes to read=4, error in (no error)=w383) -> (connection ID out=w396:refnum<k5>, data out=w395:string, error out=w398:errorcluster)  [unwired: 2 out]
            n135 = Type Cast(type=0, x=w395) -> (*(type *) &x=w394:i32)
            n136 = TCP Read(connection ID=w396, bytes to read=w394, error in (no error)=w398) -> (connection ID out=w393:refnum<k5>, data out=w390:string, error out=w392:errorcluster)  [unwired: 2 out]
            n137 = call "deleteEndString.vi"("chars to delete"=5 ("y"), "string in"=w390) -> ("substring out"=w385:string)  [unwired: 9 out]
            n138 = local read "Controls formated"() -> (w378:cluster{"name":string, "type desc":i16[]}[])
            n139 = TCP Read(connection ID=w393, bytes to read=4, error in (no error)=w392) -> (connection ID out=w381:refnum<k5>, data out=w386:string, error out=w382:errorcluster)  [unwired: 2 out]
            n140 = local read "vi reference"() -> (w377:refnum<vi>)
            n141 = call "searchElement.vi"("input"=w378, "name"=w385) -> ("output"=w389:cluster{"name":string, "type desc":i16[]})  [unwired: 9 out]
            n142 = Unbundle By Name(w389) -> ("name"=w388:string, "type desc"=w387:i16[])
            n143 = invoke class="VI" method="Ctrl Val.Set (Deprecated)"(reference=w377, "Control Name"=w388, "Type Descriptor"=w387, "Flattened Data"=w386) -> (error out=w376:errorcluster)  [unwired: 2 in, 5 out]
            n144 = call "setError.vi"("error"=w376) -> ()  [unwired: 1 out]
          }
          frame "setDouble" {
            n145 = TCP Read(connection ID=w407, bytes to read=4, error in (no error)=w406) -> (connection ID out=w420:refnum<k5>, data out=w419:string, error out=w422:errorcluster)  [unwired: 2 out]
            n146 = Type Cast(type=0, x=w419) -> (*(type *) &x=w418:i32)
            n147 = TCP Read(connection ID=w420, bytes to read=w418, error in (no error)=w422) -> (connection ID out=w417:refnum<k5>, data out=w409:string, error out=w416:errorcluster)  [unwired: 2 out]
            n148 = call "deleteEndString.vi"("chars to delete"=5 ("y"), "string in"=w409) -> ("substring out"=w408:string)  [unwired: 9 out]
            n149 = TCP Read(connection ID=w417, bytes to read=8, error in (no error)=w416) -> (connection ID out=w405:refnum<k5>, data out=w415:string, error out=w404:errorcluster)  [unwired: 2 out]
            n150 = local read "Controls formated"() -> (w402:cluster{"name":string, "type desc":i16[]}[])
            n151 = local read "vi reference"() -> (w401:refnum<vi>)
            n152 = call "searchElement.vi"("input"=w402, "name"=w408) -> ("output"=w414:cluster{"name":string, "type desc":i16[]})  [unwired: 9 out]
            n153 = Unbundle By Name(w414) -> ("name"=w413:string, "type desc"=w412:i16[])
            n154 = invoke class="VI" method="Ctrl Val.Set (Deprecated)"(reference=w401, "Control Name"=w413, "Type Descriptor"=w412, "Flattened Data"=w415) -> (error out=w400:errorcluster)  [unwired: 2 in, 5 out]
            n155 = call "setError.vi"("error"=w400) -> ()  [unwired: 1 out]
          }
          frame "setString" {
            n156 = TCP Read(connection ID=w430, bytes to read=4, error in (no error)=w429) -> (connection ID out=w450:refnum<k5>, data out=w449:string, error out=w452:errorcluster)  [unwired: 2 out]
            n157 = Type Cast(type=0, x=w449) -> (*(type *) &x=w448:i32)
            n158 = TCP Read(connection ID=w450, bytes to read=w448, error in (no error)=w452) -> (connection ID out=w447:refnum<k5>, data out=w436:string, error out=w446:errorcluster)  [unwired: 2 out]
            n159 = call "deleteEndString.vi"("chars to delete"=5, "string in"=w436) -> ("substring out"=w434:string)  [unwired: 9 out]
            n160 = local read "Controls formated"() -> (w426:cluster{"name":string, "type desc":i16[]}[])
            n161 = TCP Read(connection ID=w447, bytes to read=4, error in (no error)=w446) -> (connection ID out=w440:refnum<k5>, data out=w438:string, error out=w441:errorcluster)  [unwired: 2 out]
            n162 = Type Cast(type=0, x=w438) -> (*(type *) &x=w437:i32)
            n163 = call "searchElement.vi"("input"=w426, "name"=w434) -> ("output"=w445:cluster{"name":string, "type desc":i16[]})  [unwired: 9 out]
            n164 = local read "vi reference"() -> (w425:refnum<vi>)
            n165 = TCP Read(connection ID=w440, bytes to read=w437, error in (no error)=w441) -> (connection ID out=w427:refnum<k5>, data out=w433:string, error out=w428:errorcluster)  [unwired: 2 out]
            n166 = Variant To Flattened String(Variant=w433) -> (data string=w432:string)  [unwired: 1 out]
            n167 = Unbundle By Name(w445) -> ("name"=w444:string, "type desc"=w443:i16[])
            n168 = invoke class="VI" method="Ctrl Val.Set (Deprecated)"(reference=w425, "Control Name"=w444, "Type Descriptor"=w443, "Flattened Data"=w432) -> (error out=w424:errorcluster)  [unwired: 2 in, 5 out]
            n169 = call "setError.vi"("error"=w424) -> ()  [unwired: 1 out]
          }
          frame "setFloat" {
            n170 = TCP Read(connection ID=w461, bytes to read=4, error in (no error)=w460) -> (connection ID out=w474:refnum<k5>, data out=w473:string, error out=w476:errorcluster)  [unwired: 2 out]
            n171 = Type Cast(type=0, x=w473) -> (*(type *) &x=w472:i32)
            n172 = TCP Read(connection ID=w474, bytes to read=w472, error in (no error)=w476) -> (connection ID out=w471:refnum<k5>, data out=w463:string, error out=w470:errorcluster)  [unwired: 2 out]
            n173 = call "deleteEndString.vi"("chars to delete"=5 ("y"), "string in"=w463) -> ("substring out"=w462:string)  [unwired: 9 out]
            n174 = TCP Read(connection ID=w471, bytes to read=4, error in (no error)=w470) -> (connection ID out=w458:refnum<k5>, data out=w469:string, error out=w459:errorcluster)  [unwired: 2 out]
            n175 = local read "Controls formated"() -> (w456:cluster{"name":string, "type desc":i16[]}[])
            n176 = local read "vi reference"() -> (w455:refnum<vi>)
            n177 = call "searchElement.vi"("input"=w456, "name"=w462) -> ("output"=w468:cluster{"name":string, "type desc":i16[]})  [unwired: 9 out]
            n178 = Unbundle By Name(w468) -> ("name"=w467:string, "type desc"=w466:i16[])
            n179 = invoke class="VI" method="Ctrl Val.Set (Deprecated)"(reference=w455, "Control Name"=w467, "Type Descriptor"=w466, "Flattened Data"=w469) -> (error out=w454:errorcluster)  [unwired: 2 in, 5 out]
            n180 = call "setError.vi"("error"=w454) -> ()  [unwired: 1 out]
          }
          frame "setBooleanArray" {
            n181 = TCP Read(connection ID=w485, bytes to read=4, error in (no error)=w484) -> (connection ID out=w509:refnum<k5>, data out=w508:string, error out=w511:errorcluster)  [unwired: 2 out]
            n182 = Type Cast(type=0, x=w508) -> (*(type *) &x=w507:i32)
            n183 = TCP Read(connection ID=w509, bytes to read=w507, error in (no error)=w511) -> (connection ID out=w506:refnum<k5>, data out=w498:string, error out=w505:errorcluster)  [unwired: 2 out]
            n184 = call "deleteEndString.vi"("chars to delete"=5 ("y"), "string in"=w498) -> ("substring out"=w499:string)  [unwired: 9 out]
            n185 = TCP Read(connection ID=w506, bytes to read=4, error in (no error)=w505) -> (connection ID out=w503:refnum<k5>, data out=w501:string, error out=w504:errorcluster)  [unwired: 2 out]
            n186 = local read "Controls formated"() -> (w481:cluster{"name":string, "type desc":i16[]}[])
            n187 = Type Cast(type=0, x=w501) -> (*(type *) &x=w492:i32)
            n188 = Multiply(x=1, y=w492) -> (x*y=w494:i32)
            n189 = call "searchElement.vi"("input"=w481, "name"=w499) -> ("output"=w495:cluster{"name":string, "type desc":i16[]})  [unwired: 9 out]
            n190 = TCP Read(connection ID=w503, bytes to read=w494, error in (no error)=w504) -> (connection ID out=w482:refnum<k5>, data out=w490:string, error out=w483:errorcluster)  [unwired: 2 out]
            n191 = Unflatten From String(type=bool[] [], binary string=w490, data includes array or string size? (T)=FALSE) -> (value=w488:bool[])  [unwired: 1 in, 3 out]
            n192 = Variant To Flattened String(Variant=w488) -> (data string=w491:string)  [unwired: 1 out]
            n193 = local read "vi reference"() -> (w480:refnum<vi>)
            n194 = Unbundle By Name(w495) -> ("name"=w497:string, "type desc"=w496:i16[])
            n195 = invoke class="VI" method="Ctrl Val.Set (Deprecated)"(reference=w480, "Control Name"=w497, "Type Descriptor"=w496, "Flattened Data"=w491) -> ()  [unwired: 2 in, 6 out]
          }
          frame "setIntArray" {
            n196 = TCP Read(connection ID=w515, bytes to read=4, error in (no error)=w516) -> (connection ID out=w543:refnum<k5>, data out=w542:string, error out=w545:errorcluster)  [unwired: 2 out]
            n197 = Type Cast(type=0, x=w542) -> (*(type *) &x=w541:i32)
            n198 = TCP Read(connection ID=w543, bytes to read=w541, error in (no error)=w545) -> (connection ID out=w540:refnum<k5>, data out=w532:string, error out=w539:errorcluster)  [unwired: 2 out]
            n199 = call "deleteEndString.vi"("chars to delete"=5 ("y"), "string in"=w532) -> ("substring out"=w533:string)  [unwired: 9 out]
            n200 = TCP Read(connection ID=w540, bytes to read=4, error in (no error)=w539) -> (connection ID out=w537:refnum<k5>, data out=w535:string, error out=w538:errorcluster)  [unwired: 2 out]
            n201 = local read "Controls formated"() -> (w512:cluster{"name":string, "type desc":i16[]}[])
            n202 = Type Cast(type=0, x=w535) -> (*(type *) &x=w526:i32)
            n203 = Multiply(x=4, y=w526) -> (x*y=w528:i32)
            n204 = call "searchElement.vi"("input"=w512, "name"=w533) -> ("output"=w529:cluster{"name":string, "type desc":i16[]})  [unwired: 9 out]
            n205 = TCP Read(connection ID=w537, bytes to read=w528, error in (no error)=w538) -> (connection ID out=w518:refnum<k5>, data out=w524:string, error out=w517:errorcluster)  [unwired: 2 out]
            n206 = Unflatten From String(type=i32[] [], binary string=w524, data includes array or string size? (T)=FALSE) -> (value=w521:i32[])  [unwired: 1 in, 3 out]
            n207 = Variant To Flattened String(Variant=w521) -> (data string=w525:string)  [unwired: 1 out]
            n208 = local read "vi reference"() -> (w514:refnum<vi>)
            n209 = Unbundle By Name(w529) -> ("name"=w531:string, "type desc"=w530:i16[])
            n210 = invoke class="VI" method="Ctrl Val.Set (Deprecated)"(reference=w514, "Control Name"=w531, "Type Descriptor"=w530, "Flattened Data"=w525) -> ()  [unwired: 2 in, 6 out]
          }
          frame "setDoubleArray" {
            n211 = TCP Read(connection ID=w551, bytes to read=4, error in (no error)=w550) -> (connection ID out=w577:refnum<k5>, data out=w576:string, error out=w579:errorcluster)  [unwired: 2 out]
            n212 = Type Cast(type=0, x=w576) -> (*(type *) &x=w575:i32)
            n213 = TCP Read(connection ID=w577, bytes to read=w575, error in (no error)=w579) -> (connection ID out=w574:refnum<k5>, data out=w566:string, error out=w573:errorcluster)  [unwired: 2 out]
            n214 = call "deleteEndString.vi"("chars to delete"=5 ("y"), "string in"=w566) -> ("substring out"=w567:string)  [unwired: 9 out]
            n215 = TCP Read(connection ID=w574, bytes to read=4, error in (no error)=w573) -> (connection ID out=w571:refnum<k5>, data out=w569:string, error out=w572:errorcluster)  [unwired: 2 out]
            n216 = local read "Controls formated"() -> (w547:cluster{"name":string, "type desc":i16[]}[])
            n217 = Type Cast(type=0, x=w569) -> (*(type *) &x=w560:i32)
            n218 = Multiply(x=8, y=w560) -> (x*y=w562:i32)
            n219 = call "searchElement.vi"("input"=w547, "name"=w567) -> ("output"=w563:cluster{"name":string, "type desc":i16[]})  [unwired: 9 out]
            n220 = TCP Read(connection ID=w571, bytes to read=w562, error in (no error)=w572) -> (connection ID out=w552:refnum<k5>, data out=w558:string, error out=w549:errorcluster)  [unwired: 2 out]
            n221 = Unflatten From String(type=dbl[] [], binary string=w558, data includes array or string size? (T)=FALSE) -> (value=w555:dbl[])  [unwired: 1 in, 3 out]
            n222 = Variant To Flattened String(Variant=w555) -> (data string=w559:string)  [unwired: 1 out]
            n223 = local read "vi reference"() -> (w546:refnum<vi>)
            n224 = Unbundle By Name(w563) -> ("name"=w565:string, "type desc"=w564:i16[])
            n225 = invoke class="VI" method="Ctrl Val.Set (Deprecated)"(reference=w546, "Control Name"=w565, "Type Descriptor"=w564, "Flattened Data"=w559) -> ()  [unwired: 2 in, 6 out]
          }
          frame "setStringArray" {
            n226 = TCP Read(connection ID=w590, bytes to read=4, error in (no error)=w589) -> (connection ID out=w606:refnum<k5>, data out=w605:string, error out=w608:errorcluster)  [unwired: 2 out]
            n227 = Type Cast(type=0, x=w605) -> (*(type *) &x=w604:i32)
            n228 = TCP Read(connection ID=w606, bytes to read=w604, error in (no error)=w608) -> (connection ID out=w603:refnum<k5>, data out=w597:string, error out=w602:errorcluster)  [unwired: 2 out]
            n229 = TCP Read(connection ID=w603, bytes to read=4, error in (no error)=w602) -> (connection ID out=w584:refnum<k5>, data out=w600:string, error out=w583:errorcluster)  [unwired: 2 out]
            n230 = call "deleteEndString.vi"("chars to delete"=5 ("y"), "string in"=w597) -> ("substring out"=w598:string)  [unwired: 9 out]
            n231 = local read "Controls formated"() -> (w586:cluster{"name":string, "type desc":i16[]}[])
            n232 = Type Cast(type=0, x=w600) -> (*(type *) &x=w585:i32)
            n233 = for {
              N: w585 -> [_]
              tunnel: w584 -> [w619]
              tunnel: w583 -> [w618]
              tunnel: [w611] -> w582
              tunnel: [w610] -> w581
              tunnel: [w609] -> w580 mode=indexing
              n234 = TCP Read(connection ID=w619, bytes to read=4, error in (no error)=w618) -> (connection ID out=w616:refnum<k5>, data out=w613:string, error out=w615:errorcluster)  [unwired: 2 out]
              n235 = Type Cast(type=0, x=w613) -> (*(type *) &x=w612:i32)
              n236 = TCP Read(connection ID=w616, bytes to read=w612, error in (no error)=w615) -> (connection ID out=w611:refnum<k5>, data out=w609:string, error out=w610:errorcluster)  [unwired: 2 out]
            }
            n237 = call "searchElement.vi"("input"=w586, "name"=w598) -> ("output"=w594:cluster{"name":string, "type desc":i16[]})  [unwired: 9 out]
            n238 = Variant To Flattened String(Variant=w580) -> (data string=w593:string)  [unwired: 1 out]
            n239 = local read "vi reference"() -> (w587:refnum<vi>)
            n240 = Unbundle By Name(w594) -> ("name"=w596:string, "type desc"=w595:i16[])
            n241 = invoke class="VI" method="Ctrl Val.Set (Deprecated)"(reference=w587, "Control Name"=w596, "Type Descriptor"=w595, "Flattened Data"=w593) -> ()  [unwired: 2 in, 6 out]
          }
          frame "setFloatArray" {
            n242 = TCP Read(connection ID=w623, bytes to read=4, error in (no error)=w622) -> (connection ID out=w651:refnum<k5>, data out=w650:string, error out=w653:errorcluster)  [unwired: 2 out]
            n243 = Type Cast(type=0, x=w650) -> (*(type *) &x=w649:i32)
            n244 = TCP Read(connection ID=w651, bytes to read=w649, error in (no error)=w653) -> (connection ID out=w648:refnum<k5>, data out=w640:string, error out=w647:errorcluster)  [unwired: 2 out]
            n245 = call "deleteEndString.vi"("chars to delete"=5 ("y"), "string in"=w640) -> ("substring out"=w641:string)  [unwired: 9 out]
            n246 = TCP Read(connection ID=w648, bytes to read=4, error in (no error)=w647) -> (connection ID out=w645:refnum<k5>, data out=w643:string, error out=w646:errorcluster)  [unwired: 2 out]
            n247 = local read "Controls formated"() -> (w621:cluster{"name":string, "type desc":i16[]}[])
            n248 = Type Cast(type=0, x=w643) -> (*(type *) &x=w634:i32)
            n249 = Multiply(x=4, y=w634) -> (x*y=w636:i32)
            n250 = call "searchElement.vi"("input"=w621, "name"=w641) -> ("output"=w637:cluster{"name":string, "type desc":i16[]})  [unwired: 9 out]
            n251 = TCP Read(connection ID=w645, bytes to read=w636, error in (no error)=w646) -> (connection ID out=w624:refnum<k5>, data out=w632:string, error out=w625:errorcluster)  [unwired: 2 out]
            n252 = Unflatten From String(type=sgl[] [], binary string=w632, data includes array or string size? (T)=FALSE) -> (value=w629:sgl[])  [unwired: 1 in, 3 out]
            n253 = local read "vi reference"() -> (w620:refnum<vi>)
            n254 = Variant To Flattened String(Variant=w629) -> (data string=w633:string)  [unwired: 1 out]
            n255 = Unbundle By Name(w637) -> ("name"=w639:string, "type desc"=w638:i16[])
            n256 = invoke class="VI" method="Ctrl Val.Set (Deprecated)"(reference=w620, "Control Name"=w639, "Type Descriptor"=w638, "Flattened Data"=w633) -> ()  [unwired: 2 in, 6 out]
          }
          frame "setBooleanArray2D" {
            w679 = 4 ("bytes to read")
            n257 = TCP Read(connection ID=w661, bytes to read=4, error in (no error)=w660) -> (connection ID out=w689:refnum<k5>, data out=w688:string, error out=w691:errorcluster)  [unwired: 2 out]
            n258 = Type Cast(type=0, x=w688) -> (*(type *) &x=w687:i32)
            n259 = TCP Read(connection ID=w689, bytes to read=w687, error in (no error)=w691) -> (connection ID out=w686:refnum<k5>, data out=w680:string, error out=w685:errorcluster)  [unwired: 2 out]
            n260 = call "deleteEndString.vi"("chars to delete"=5 ("y"), "string in"=w680) -> ("substring out"=w681:string)  [unwired: 9 out]
            n261 = local read "Controls formated"() -> (w656:cluster{"name":string, "type desc":i16[]}[])
            n262 = TCP Read(connection ID=w686, bytes to read=w679, error in (no error)=w685) -> (connection ID out=w683:refnum<k5>, data out=w678:string, error out=w684:errorcluster)  [unwired: 2 out]
            n263 = Type Cast(type=0, x=w678) -> (*(type *) &x=w672:i32)
            n264 = TCP Read(connection ID=w683, bytes to read=w679, error in (no error)=w684) -> (connection ID out=w675:refnum<k5>, data out=w676:string, error out=w674:errorcluster)  [unwired: 2 out]
            n265 = call "searchElement.vi"("input"=w656, "name"=w681) -> ("output"=w668:cluster{"name":string, "type desc":i16[]})  [unwired: 9 out]
            n266 = Type Cast(type=0, x=w676) -> (*(type *) &x=w673:i32)
            n267 = Compound Arithmetic op=MULTIPLY(w672, w673, 1 ("value")) -> (w671:i32)
            n268 = TCP Read(connection ID=w675, bytes to read=w671, error in (no error)=w674) -> (connection ID out=w659:refnum<k5>, data out=w666:string, error out=w658:errorcluster)  [unwired: 2 out]
            n269 = Unflatten From String(type=bool[][] [], binary string=w666, data includes array or string size? (T)=FALSE) -> (value=w665:bool[][])  [unwired: 1 in, 3 out]
            n270 = Variant To Flattened String(Variant=w665) -> (data string=w664:string)  [unwired: 1 out]
            n271 = local read "vi reference"() -> (w655:refnum<vi>)
            n272 = Unbundle By Name(w668) -> ("name"=w670:string, "type desc"=w669:i16[])
            n273 = invoke class="VI" method="Ctrl Val.Set (Deprecated)"(reference=w655, "Control Name"=w670, "Type Descriptor"=w669, "Flattened Data"=w664) -> ()  [unwired: 2 in, 6 out]
          }
          frame "setIntArray2D" {
            w718 = 4 ("bytes to read")
            n274 = TCP Read(connection ID=w700, bytes to read=4, error in (no error)=w699) -> (connection ID out=w728:refnum<k5>, data out=w727:string, error out=w730:errorcluster)  [unwired: 2 out]
            n275 = Type Cast(type=0, x=w727) -> (*(type *) &x=w726:i32)
            n276 = TCP Read(connection ID=w728, bytes to read=w726, error in (no error)=w730) -> (connection ID out=w725:refnum<k5>, data out=w719:string, error out=w724:errorcluster)  [unwired: 2 out]
            n277 = call "deleteEndString.vi"("chars to delete"=5 ("y"), "string in"=w719) -> ("substring out"=w720:string)  [unwired: 9 out]
            n278 = local read "Controls formated"() -> (w693:cluster{"name":string, "type desc":i16[]}[])
            n279 = TCP Read(connection ID=w725, bytes to read=w718, error in (no error)=w724) -> (connection ID out=w722:refnum<k5>, data out=w717:string, error out=w723:errorcluster)  [unwired: 2 out]
            n280 = Type Cast(type=0, x=w717) -> (*(type *) &x=w711:i32)
            n281 = TCP Read(connection ID=w722, bytes to read=w718, error in (no error)=w723) -> (connection ID out=w714:refnum<k5>, data out=w715:string, error out=w713:errorcluster)  [unwired: 2 out]
            n282 = call "searchElement.vi"("input"=w693, "name"=w720) -> ("output"=w707:cluster{"name":string, "type desc":i16[]})  [unwired: 9 out]
            n283 = Type Cast(type=0, x=w715) -> (*(type *) &x=w712:i32)
            n284 = Compound Arithmetic op=MULTIPLY(w711, w712, 4 ("value")) -> (w710:i32)
            n285 = TCP Read(connection ID=w714, bytes to read=w710, error in (no error)=w713) -> (connection ID out=w698:refnum<k5>, data out=w705:string, error out=w697:errorcluster)  [unwired: 2 out]
            n286 = Unflatten From String(type=i32[][] [], binary string=w705, data includes array or string size? (T)=FALSE) -> (value=w704:i32[][])  [unwired: 1 in, 3 out]
            n287 = Variant To Flattened String(Variant=w704) -> (data string=w703:string)  [unwired: 1 out]
            n288 = local read "vi reference"() -> (w694:refnum<vi>)
            n289 = Unbundle By Name(w707) -> ("name"=w709:string, "type desc"=w708:i16[])
            n290 = invoke class="VI" method="Ctrl Val.Set (Deprecated)"(reference=w694, "Control Name"=w709, "Type Descriptor"=w708, "Flattened Data"=w703) -> ()  [unwired: 2 in, 6 out]
          }
          frame "setDoubleArray2D" {
            w757 = 4 ("bytes to read")
            n291 = TCP Read(connection ID=w739, bytes to read=4, error in (no error)=w738) -> (connection ID out=w767:refnum<k5>, data out=w766:string, error out=w769:errorcluster)  [unwired: 2 out]
            n292 = Type Cast(type=0, x=w766) -> (*(type *) &x=w765:i32)
            n293 = TCP Read(connection ID=w767, bytes to read=w765, error in (no error)=w769) -> (connection ID out=w764:refnum<k5>, data out=w758:string, error out=w763:errorcluster)  [unwired: 2 out]
            n294 = call "deleteEndString.vi"("chars to delete"=5 ("y"), "string in"=w758) -> ("substring out"=w759:string)  [unwired: 9 out]
            n295 = local read "Controls formated"() -> (w732:cluster{"name":string, "type desc":i16[]}[])
            n296 = TCP Read(connection ID=w764, bytes to read=w757, error in (no error)=w763) -> (connection ID out=w761:refnum<k5>, data out=w756:string, error out=w762:errorcluster)  [unwired: 2 out]
            n297 = Type Cast(type=0, x=w756) -> (*(type *) &x=w750:i32)
            n298 = TCP Read(connection ID=w761, bytes to read=w757, error in (no error)=w762) -> (connection ID out=w753:refnum<k5>, data out=w754:string, error out=w752:errorcluster)  [unwired: 2 out]
            n299 = call "searchElement.vi"("input"=w732, "name"=w759) -> ("output"=w746:cluster{"name":string, "type desc":i16[]})  [unwired: 9 out]
            n300 = Type Cast(type=0, x=w754) -> (*(type *) &x=w751:i32)
            n301 = Compound Arithmetic op=MULTIPLY(w750, w751, 8 ("value")) -> (w749:i32)
            n302 = TCP Read(connection ID=w753, bytes to read=w749, error in (no error)=w752) -> (connection ID out=w736:refnum<k5>, data out=w744:string, error out=w737:errorcluster)  [unwired: 2 out]
            n303 = Unflatten From String(type=dbl[][] [], binary string=w744, data includes array or string size? (T)=FALSE) -> (value=w742:dbl[][])  [unwired: 1 in, 3 out]
            n304 = local read "vi reference"() -> (w733:refnum<vi>)
            n305 = Variant To Flattened String(Variant=w742) -> (data string=w741:string)  [unwired: 1 out]
            n306 = Unbundle By Name(w746) -> ("name"=w748:string, "type desc"=w747:i16[])
            n307 = invoke class="VI" method="Ctrl Val.Set (Deprecated)"(reference=w733, "Control Name"=w748, "Type Descriptor"=w747, "Flattened Data"=w741) -> ()  [unwired: 2 in, 6 out]
          }
          frame "setStringArray2D" {
            w791 = 4 ("bytes to read")
            n308 = TCP Read(connection ID=w780, bytes to read=4, error in (no error)=w779) -> (connection ID out=w801:refnum<k5>, data out=w800:string, error out=w803:errorcluster)  [unwired: 2 out]
            n309 = Type Cast(type=0, x=w800) -> (*(type *) &x=w799:i32)
            n310 = TCP Read(connection ID=w801, bytes to read=w799, error in (no error)=w803) -> (connection ID out=w798:refnum<k5>, data out=w792:string, error out=w797:errorcluster)  [unwired: 2 out]
            n311 = TCP Read(connection ID=w798, bytes to read=w791, error in (no error)=w797) -> (connection ID out=w795:refnum<k5>, data out=w790:string, error out=w796:errorcluster)  [unwired: 2 out]
            n312 = call "deleteEndString.vi"("chars to delete"=5 ("y"), "string in"=w792) -> ("substring out"=w793:string)  [unwired: 9 out]
            n313 = local read "Controls formated"() -> (w782:cluster{"name":string, "type desc":i16[]}[])
            n314 = Type Cast(type=0, x=w790) -> (*(type *) &x=w778:i32)
            n315 = TCP Read(connection ID=w795, bytes to read=w791, error in (no error)=w796) -> (connection ID out=w776:refnum<k5>, data out=w788:string, error out=w775:errorcluster)  [unwired: 2 out]
            n316 = call "searchElement.vi"("input"=w782, "name"=w793) -> ("output"=w785:cluster{"name":string, "type desc":i16[]})  [unwired: 9 out]
            n317 = Type Cast(type=0, x=w788) -> (*(type *) &x=w777:i32)
            n318 = for {
              N: w778 -> [_]
              tunnel: w777 -> [w810]
              tunnel: w776 -> [w809]
              tunnel: w775 -> [w808]
              tunnel: [w807] -> w774
              tunnel: [w806] -> w773
              tunnel: [w805] -> w771 mode=indexing
              n319 = for {
                N: w810 -> [_]
                tunnel: w809 -> [w820]
                tunnel: w808 -> [w819]
                tunnel: [w816] -> w807
                tunnel: [w815] -> w806
                tunnel: [w811] -> w805 mode=indexing
                n320 = TCP Read(connection ID=w820, error in (no error)=w819) -> (connection ID out=w818:refnum<k5>, data out=w813:string, error out=w817:errorcluster)  [unwired: 3 out]
                n321 = Type Cast(type=0, x=w813) -> (*(type *) &x=w812:i32)
                n322 = TCP Read(connection ID=w818, bytes to read=w812, error in (no error)=w817) -> (connection ID out=w816:refnum<k5>, data out=w811:string, error out=w815:errorcluster)  [unwired: 2 out]
              }
            }
            n323 = Variant To Flattened String(Variant=w771) -> (data string=w784:string)  [unwired: 1 out]
            n324 = local read "vi reference"() -> (w781:refnum<vi>)
            n325 = Unbundle By Name(w785) -> ("name"=w787:string, "type desc"=w786:i16[])
            n326 = invoke class="VI" method="Ctrl Val.Set (Deprecated)"(reference=w781, "Control Name"=w787, "Type Descriptor"=w786, "Flattened Data"=w784) -> ()  [unwired: 2 in, 6 out]
          }
          frame "setFloatArray2D" {
            w846 = 4 ("bytes to read")
            n327 = TCP Read(connection ID=w827, bytes to read=4, error in (no error)=w826) -> (connection ID out=w856:refnum<k5>, data out=w855:string, error out=w858:errorcluster)  [unwired: 2 out]
            n328 = Type Cast(type=0, x=w855) -> (*(type *) &x=w854:i32)
            n329 = TCP Read(connection ID=w856, bytes to read=w854, error in (no error)=w858) -> (connection ID out=w853:refnum<k5>, data out=w847:string, error out=w852:errorcluster)  [unwired: 2 out]
            n330 = call "deleteEndString.vi"("chars to delete"=5 ("y"), "string in"=w847) -> ("substring out"=w848:string)  [unwired: 9 out]
            n331 = local read "Controls formated"() -> (w821:cluster{"name":string, "type desc":i16[]}[])
            n332 = TCP Read(connection ID=w853, bytes to read=w846, error in (no error)=w852) -> (connection ID out=w850:refnum<k5>, data out=w845:string, error out=w851:errorcluster)  [unwired: 2 out]
            n333 = Type Cast(type=0, x=w845) -> (*(type *) &x=w839:i32)
            n334 = TCP Read(connection ID=w850, bytes to read=w846, error in (no error)=w851) -> (connection ID out=w842:refnum<k5>, data out=w843:string, error out=w841:errorcluster)  [unwired: 2 out]
            n335 = call "searchElement.vi"("input"=w821, "name"=w848) -> ("output"=w835:cluster{"name":string, "type desc":i16[]})  [unwired: 9 out]
            n336 = Type Cast(type=0, x=w843) -> (*(type *) &x=w840:i32)
            n337 = Compound Arithmetic op=MULTIPLY(w839, w840, 4 ("value")) -> (w838:i32)
            n338 = TCP Read(connection ID=w842, bytes to read=w838, error in (no error)=w841) -> (connection ID out=w824:refnum<k5>, data out=w833:string, error out=w825:errorcluster)  [unwired: 2 out]
            n339 = Unflatten From String(type=sgl[][] [], binary string=w833, data includes array or string size? (T)=FALSE) -> (value=w831:sgl[][])  [unwired: 1 in, 3 out]
            n340 = Variant To Flattened String(Variant=w831) -> (data string=w830:string)  [unwired: 1 out]
            n341 = local read "vi reference"() -> (w822:refnum<vi>)
            n342 = Unbundle By Name(w835) -> ("name"=w837:string, "type desc"=w836:i16[])
            n343 = invoke class="VI" method="Ctrl Val.Set (Deprecated)"(reference=w822, "Control Name"=w837, "Type Descriptor"=w836, "Flattened Data"=w830) -> ()  [unwired: 2 in, 6 out]
          }
          frame "getBoolean" {
            n344 = TCP Read(connection ID=w871, bytes to read=4, error in (no error)=w870) -> (connection ID out=w875:refnum<k5>, data out=w878:string, error out=w874:errorcluster)  [unwired: 2 out]
            n345 = Type Cast(type=0, x=w878) -> (*(type *) &x=w876:i32)
            n346 = TCP Read(connection ID=w875, bytes to read=w876, error in (no error)=w874) -> (connection ID out=w867:refnum<k5>, data out=w873:string, error out=w866:errorcluster)  [unwired: 2 out]
            n347 = local read "Indicators formated"() -> (w868:cluster{"name":string, "type desc":i16[]}[])
            n348 = call "deleteEndString.vi"("chars to delete"=5, "string in"=w873) -> ("substring out"=w872:string)  [unwired: 9 out]
            n349 = local read "vi reference"() -> (w861:refnum<vi>)
            n350 = call "searchElement.vi"("input"=w868, "name"=w872) -> ("output"=w880:cluster{"name":string, "type desc":i16[]})  [unwired: 9 out]
            n351 = Unbundle By Name(w880) -> ("name"=w879:string)
            n352 = invoke class="VI" method="Ctrl Val.Get (Deprecated)"(reference=w861, "Control Name"=w879) -> (error out=w860:errorcluster, "Get Control Value"=w862:string)  [unwired: 3 in, 3 out]
            n353 = TCP Write(connection ID=w867, data in=w862, error in (no error)=w866) -> (connection ID out=w863:refnum<k5>, error out=w865:errorcluster)  [unwired: 2 out]
            n354 = call "setError.vi"("error"=w860) -> ()  [unwired: 1 out]
          }
          frame "getInt" {
            n355 = TCP Read(connection ID=w890, bytes to read=4, error in (no error)=w889) -> (connection ID out=w897:refnum<k5>, data out=w900:string, error out=w896:errorcluster)  [unwired: 2 out]
            n356 = Type Cast(type=0, x=w900) -> (*(type *) &x=w898:i32)
            n357 = TCP Read(connection ID=w897, bytes to read=w898, error in (no error)=w896) -> (connection ID out=w892:refnum<k5>, data out=w895:string, error out=w891:errorcluster)  [unwired: 2 out]
            n358 = local read "Indicators formated"() -> (w884:cluster{"name":string, "type desc":i16[]}[])
            n359 = call "deleteEndString.vi"("chars to delete"=5, "string in"=w895) -> ("substring out"=w894:string)  [unwired: 9 out]
            n360 = local read "vi reference"() -> (w883:refnum<vi>)
            n361 = call "searchElement.vi"("input"=w884, "name"=w894) -> ("output"=w902:cluster{"name":string, "type desc":i16[]})  [unwired: 9 out]
            n362 = Unbundle By Name(w902) -> ("name"=w901:string)
            n363 = invoke class="VI" method="Ctrl Val.Get (Deprecated)"(reference=w883, "Control Name"=w901) -> (error out=w882:errorcluster, "Get Control Value"=w886:string)  [unwired: 3 in, 3 out]
            n364 = TCP Write(connection ID=w892, data in=w886, error in (no error)=w891) -> (connection ID out=w887:refnum<k5>, error out=w888:errorcluster)  [unwired: 2 out]
            n365 = call "setError.vi"("error"=w882) -> ()  [unwired: 1 out]
          }
          frame "getDouble" {
            n366 = TCP Read(connection ID=w912, bytes to read=4, error in (no error)=w911) -> (connection ID out=w919:refnum<k5>, data out=w922:string, error out=w918:errorcluster)  [unwired: 2 out]
            n367 = Type Cast(type=0, x=w922) -> (*(type *) &x=w920:i32)
            n368 = TCP Read(connection ID=w919, bytes to read=w920, error in (no error)=w918) -> (connection ID out=w914:refnum<k5>, data out=w917:string, error out=w913:errorcluster)  [unwired: 2 out]
            n369 = call "deleteEndString.vi"("chars to delete"=5, "string in"=w917) -> ("substring out"=w916:string)  [unwired: 9 out]
            n370 = local read "Indicators formated"() -> (w905:cluster{"name":string, "type desc":i16[]}[])
            n371 = local read "vi reference"() -> (w906:refnum<vi>)
            n372 = call "searchElement.vi"("input"=w905, "name"=w916) -> ("output"=w924:cluster{"name":string, "type desc":i16[]})  [unwired: 9 out]
            n373 = Unbundle By Name(w924) -> ("name"=w923:string)
            n374 = invoke class="VI" method="Ctrl Val.Get (Deprecated)"(reference=w906, "Control Name"=w923) -> (error out=w904:errorcluster, "Get Control Value"=w907:string)  [unwired: 3 in, 3 out]
            n375 = TCP Write(connection ID=w914, data in=w907, error in (no error)=w913) -> (connection ID out=w909:refnum<k5>, error out=w910:errorcluster)  [unwired: 2 out]
            n376 = call "setError.vi"("error"=w904) -> ()  [unwired: 1 out]
          }
          frame "getString" {
            n377 = TCP Read(connection ID=w934, bytes to read=4, error in (no error)=w933) -> (connection ID out=w941:refnum<k5>, data out=w944:string, error out=w940:errorcluster)  [unwired: 2 out]
            n378 = Type Cast(type=0, x=w944) -> (*(type *) &x=w942:i32)
            n379 = TCP Read(connection ID=w941, bytes to read=w942, error in (no error)=w940) -> (connection ID out=w936:refnum<k5>, data out=w939:string, error out=w935:errorcluster)  [unwired: 2 out]
            n380 = call "deleteEndString.vi"("chars to delete"=5, "string in"=w939) -> ("substring out"=w938:string)  [unwired: 9 out]
            n381 = local read "Indicators formated"() -> (w927:cluster{"name":string, "type desc":i16[]}[])
            n382 = call "searchElement.vi"("input"=w927, "name"=w938) -> ("output"=w946:cluster{"name":string, "type desc":i16[]})  [unwired: 9 out]
            n383 = local read "vi reference"() -> (w928:refnum<vi>)
            n384 = Unbundle By Name(w946) -> ("name"=w945:string)
            n385 = invoke class="VI" method="Ctrl Val.Get (Deprecated)"(reference=w928, "Control Name"=w945) -> (error out=w926:errorcluster, "Get Control Value"=w930:string)  [unwired: 3 in, 3 out]
            n386 = TCP Write(connection ID=w936, data in=w930, error in (no error)=w935) -> (connection ID out=w931:refnum<k5>, error out=w932:errorcluster)  [unwired: 2 out]
            n387 = call "setError.vi"("error"=w926) -> ()  [unwired: 1 out]
          }
          frame "getFloat" {
            n388 = TCP Read(connection ID=w955, bytes to read=4, error in (no error)=w954) -> (connection ID out=w963:refnum<k5>, data out=w966:string, error out=w962:errorcluster)  [unwired: 2 out]
            n389 = Type Cast(type=0, x=w966) -> (*(type *) &x=w964:i32)
            n390 = TCP Read(connection ID=w963, bytes to read=w964, error in (no error)=w962) -> (connection ID out=w958:refnum<k5>, data out=w961:string, error out=w957:errorcluster)  [unwired: 2 out]
            n391 = call "deleteEndString.vi"("chars to delete"=5, "string in"=w961) -> ("substring out"=w960:string)  [unwired: 9 out]
            n392 = local read "Controls formated"() -> (w949:cluster{"name":string, "type desc":i16[]}[])
            n393 = local read "vi reference"() -> (w950:refnum<vi>)
            n394 = call "searchElement.vi"("input"=w949, "name"=w960) -> ("output"=w968:cluster{"name":string, "type desc":i16[]})  [unwired: 9 out]
            n395 = Unbundle By Name(w968) -> ("name"=w967:string)
            n396 = invoke class="VI" method="Ctrl Val.Get (Deprecated)"(reference=w950, "Control Name"=w967) -> (error out=w948:errorcluster, "Get Control Value"=w956:string)  [unwired: 3 in, 3 out]
            n397 = TCP Write(connection ID=w958, data in=w956, error in (no error)=w957) -> (connection ID out=w952:refnum<k5>, error out=w953:errorcluster)  [unwired: 2 out]
            n398 = call "setError.vi"("error"=w948) -> ()  [unwired: 1 out]
          }
          frame "getBooleanArray" {
            n399 = TCP Read(connection ID=w978, bytes to read=4, error in (no error)=w977) -> (connection ID out=w985:refnum<k5>, data out=w988:string, error out=w984:errorcluster)  [unwired: 2 out]
            n400 = Type Cast(type=0, x=w988) -> (*(type *) &x=w986:i32)
            n401 = TCP Read(connection ID=w985, bytes to read=w986, error in (no error)=w984) -> (connection ID out=w980:refnum<k5>, data out=w983:string, error out=w979:errorcluster)  [unwired: 2 out]
            n402 = call "deleteEndString.vi"("chars to delete"=5, "string in"=w983) -> ("substring out"=w982:string)  [unwired: 9 out]
            n403 = local read "Indicators formated"() -> (w973:cluster{"name":string, "type desc":i16[]}[])
            n404 = local read "vi reference"() -> (w972:refnum<vi>)
            n405 = call "searchElement.vi"("input"=w973, "name"=w982) -> ("output"=w990:cluster{"name":string, "type desc":i16[]})  [unwired: 9 out]
            n406 = Unbundle By Name(w990) -> ("name"=w989:string)
            n407 = invoke class="VI" method="Ctrl Val.Get (Deprecated)"(reference=w972, "Control Name"=w989) -> (error out=w970:errorcluster, "Get Control Value"=w974:string)  [unwired: 3 in, 3 out]
            n408 = TCP Write(connection ID=w980, data in=w974, error in (no error)=w979) -> (connection ID out=w975:refnum<k5>, error out=w976:errorcluster)  [unwired: 2 out]
            n409 = call "setError.vi"("error"=w970) -> ()  [unwired: 1 out]
          }
          frame "getIntArray" {
            n410 = TCP Read(connection ID=w1000, bytes to read=4, error in (no error)=w999) -> (connection ID out=w1007:refnum<k5>, data out=w1010:string, error out=w1006:errorcluster)  [unwired: 2 out]
            n411 = Type Cast(type=0, x=w1010) -> (*(type *) &x=w1008:i32)
            n412 = TCP Read(connection ID=w1007, bytes to read=w1008, error in (no error)=w1006) -> (connection ID out=w1002:refnum<k5>, data out=w1005:string, error out=w1001:errorcluster)  [unwired: 2 out]
            n413 = call "deleteEndString.vi"("chars to delete"=5, "string in"=w1005) -> ("substring out"=w1004:string)  [unwired: 9 out]
            n414 = local read "Indicators formated"() -> (w994:cluster{"name":string, "type desc":i16[]}[])
            n415 = local read "vi reference"() -> (w993:refnum<vi>)
            n416 = call "searchElement.vi"("input"=w994, "name"=w1004) -> ("output"=w1012:cluster{"name":string, "type desc":i16[]})  [unwired: 9 out]
            n417 = Unbundle By Name(w1012) -> ("name"=w1011:string)
            n418 = invoke class="VI" method="Ctrl Val.Get (Deprecated)"(reference=w993, "Control Name"=w1011) -> (error out=w992:errorcluster, "Get Control Value"=w995:string)  [unwired: 3 in, 3 out]
            n419 = TCP Write(connection ID=w1002, data in=w995, error in (no error)=w1001) -> (connection ID out=w997:refnum<k5>, error out=w998:errorcluster)  [unwired: 2 out]
            n420 = call "setError.vi"("error"=w992) -> ()  [unwired: 1 out]
          }
          frame "getDoubleArray" {
            n421 = TCP Read(connection ID=w1022, bytes to read=4, error in (no error)=w1021) -> (connection ID out=w1029:refnum<k5>, data out=w1032:string, error out=w1028:errorcluster)  [unwired: 2 out]
            n422 = Type Cast(type=0, x=w1032) -> (*(type *) &x=w1030:i32)
            n423 = TCP Read(connection ID=w1029, bytes to read=w1030, error in (no error)=w1028) -> (connection ID out=w1024:refnum<k5>, data out=w1027:string, error out=w1023:errorcluster)  [unwired: 2 out]
            n424 = call "deleteEndString.vi"("chars to delete"=5, "string in"=w1027) -> ("substring out"=w1026:string)  [unwired: 9 out]
            n425 = local read "Indicators formated"() -> (w1015:cluster{"name":string, "type desc":i16[]}[])
            n426 = call "searchElement.vi"("input"=w1015, "name"=w1026) -> ("output"=w1034:cluster{"name":string, "type desc":i16[]})  [unwired: 9 out]
            n427 = local read "vi reference"() -> (w1016:refnum<vi>)
            n428 = Unbundle By Name(w1034) -> ("name"=w1033:string)
            n429 = invoke class="VI" method="Ctrl Val.Get (Deprecated)"(reference=w1016, "Control Name"=w1033) -> (error out=w1014:errorcluster, "Get Control Value"=w1017:string)  [unwired: 3 in, 3 out]
            n430 = TCP Write(connection ID=w1024, data in=w1017, error in (no error)=w1023) -> (connection ID out=w1019:refnum<k5>, error out=w1020:errorcluster)  [unwired: 2 out]
            n431 = call "setError.vi"("error"=w1014) -> ()  [unwired: 1 out]
          }
          frame "getStringArray" {
            n432 = TCP Read(connection ID=w1044, bytes to read=4, error in (no error)=w1043) -> (connection ID out=w1051:refnum<k5>, data out=w1054:string, error out=w1050:errorcluster)  [unwired: 2 out]
            n433 = Type Cast(type=0, x=w1054) -> (*(type *) &x=w1052:i32)
            n434 = TCP Read(connection ID=w1051, bytes to read=w1052, error in (no error)=w1050) -> (connection ID out=w1046:refnum<k5>, data out=w1049:string, error out=w1045:errorcluster)  [unwired: 2 out]
            n435 = call "deleteEndString.vi"("chars to delete"=5, "string in"=w1049) -> ("substring out"=w1048:string)  [unwired: 9 out]
            n436 = local read "Indicators formated"() -> (w1038:cluster{"name":string, "type desc":i16[]}[])
            n437 = call "searchElement.vi"("input"=w1038, "name"=w1048) -> ("output"=w1056:cluster{"name":string, "type desc":i16[]})  [unwired: 9 out]
            n438 = local read "vi reference"() -> (w1037:refnum<vi>)
            n439 = Unbundle By Name(w1056) -> ("name"=w1055:string)
            n440 = invoke class="VI" method="Ctrl Val.Get (Deprecated)"(reference=w1037, "Control Name"=w1055) -> (error out=w1036:errorcluster, "Get Control Value"=w1040:string)  [unwired: 3 in, 3 out]
            n441 = TCP Write(connection ID=w1046, data in=w1040, error in (no error)=w1045) -> (connection ID out=w1041:refnum<k5>, error out=w1042:errorcluster)  [unwired: 2 out]
            n442 = call "setError.vi"("error"=w1036) -> ()  [unwired: 1 out]
          }
          frame "getFloatArray" {
            n443 = TCP Read(connection ID=w1065, bytes to read=4, error in (no error)=w1064) -> (connection ID out=w1073:refnum<k5>, data out=w1076:string, error out=w1072:errorcluster)  [unwired: 2 out]
            n444 = Type Cast(type=0, x=w1076) -> (*(type *) &x=w1074:i32)
            n445 = TCP Read(connection ID=w1073, bytes to read=w1074, error in (no error)=w1072) -> (connection ID out=w1068:refnum<k5>, data out=w1071:string, error out=w1067:errorcluster)  [unwired: 2 out]
            n446 = call "deleteEndString.vi"("chars to delete"=5, "string in"=w1071) -> ("substring out"=w1070:string)  [unwired: 9 out]
            n447 = local read "Controls formated"() -> (w1059:cluster{"name":string, "type desc":i16[]}[])
            n448 = local read "vi reference"() -> (w1060:refnum<vi>)
            n449 = call "searchElement.vi"("input"=w1059, "name"=w1070) -> ("output"=w1078:cluster{"name":string, "type desc":i16[]})  [unwired: 9 out]
            n450 = Unbundle By Name(w1078) -> ("name"=w1077:string)
            n451 = invoke class="VI" method="Ctrl Val.Get (Deprecated)"(reference=w1060, "Control Name"=w1077) -> (error out=w1058:errorcluster, "Get Control Value"=w1066:string)  [unwired: 3 in, 3 out]
            n452 = TCP Write(connection ID=w1068, data in=w1066, error in (no error)=w1067) -> (connection ID out=w1063:refnum<k5>, error out=w1062:errorcluster)  [unwired: 2 out]
            n453 = call "setError.vi"("error"=w1058) -> ()  [unwired: 1 out]
          }
          frame "getBooleanArray2D" {
            n454 = TCP Read(connection ID=w1088, bytes to read=4, error in (no error)=w1087) -> (connection ID out=w1095:refnum<k5>, data out=w1098:string, error out=w1094:errorcluster)  [unwired: 2 out]
            n455 = Type Cast(type=0, x=w1098) -> (*(type *) &x=w1096:i32)
            n456 = TCP Read(connection ID=w1095, bytes to read=w1096, error in (no error)=w1094) -> (connection ID out=w1090:refnum<k5>, data out=w1093:string, error out=w1089:errorcluster)  [unwired: 2 out]
            n457 = call "deleteEndString.vi"("chars to delete"=5, "string in"=w1093) -> ("substring out"=w1092:string)  [unwired: 9 out]
            n458 = local read "Indicators formated"() -> (w1082:cluster{"name":string, "type desc":i16[]}[])
            n459 = call "searchElement.vi"("input"=w1082, "name"=w1092) -> ("output"=w1100:cluster{"name":string, "type desc":i16[]})  [unwired: 9 out]
            n460 = local read "vi reference"() -> (w1081:refnum<vi>)
            n461 = Unbundle By Name(w1100) -> ("name"=w1099:string)
            n462 = invoke class="VI" method="Ctrl Val.Get (Deprecated)"(reference=w1081, "Control Name"=w1099) -> (error out=w1080:errorcluster, "Get Control Value"=w1084:string)  [unwired: 3 in, 3 out]
            n463 = TCP Write(connection ID=w1090, data in=w1084, error in (no error)=w1089) -> (connection ID out=w1086:refnum<k5>, error out=w1085:errorcluster)  [unwired: 2 out]
            n464 = call "setError.vi"("error"=w1080) -> ()  [unwired: 1 out]
          }
          frame "getIntArray2D" {
            n465 = TCP Read(connection ID=w1110, bytes to read=4, error in (no error)=w1109) -> (connection ID out=w1117:refnum<k5>, data out=w1120:string, error out=w1116:errorcluster)  [unwired: 2 out]
            n466 = Type Cast(type=0, x=w1120) -> (*(type *) &x=w1118:i32)
            n467 = TCP Read(connection ID=w1117, bytes to read=w1118, error in (no error)=w1116) -> (connection ID out=w1112:refnum<k5>, data out=w1115:string, error out=w1111:errorcluster)  [unwired: 2 out]
            n468 = local read "Indicators formated"() -> (w1104:cluster{"name":string, "type desc":i16[]}[])
            n469 = call "deleteEndString.vi"("chars to delete"=5, "string in"=w1115) -> ("substring out"=w1114:string)  [unwired: 9 out]
            n470 = local read "vi reference"() -> (w1103:refnum<vi>)
            n471 = call "searchElement.vi"("input"=w1104, "name"=w1114) -> ("output"=w1122:cluster{"name":string, "type desc":i16[]})  [unwired: 9 out]
            n472 = Unbundle By Name(w1122) -> ("name"=w1121:string)
            n473 = invoke class="VI" method="Ctrl Val.Get (Deprecated)"(reference=w1103, "Control Name"=w1121) -> (error out=w1102:errorcluster, "Get Control Value"=w1106:string)  [unwired: 3 in, 3 out]
            n474 = TCP Write(connection ID=w1112, data in=w1106, error in (no error)=w1111) -> (connection ID out=w1107:refnum<k5>, error out=w1108:errorcluster)  [unwired: 2 out]
            n475 = call "setError.vi"("error"=w1102) -> ()  [unwired: 1 out]
          }
          frame "getDoubleArray2D" {
            n476 = TCP Read(connection ID=w1132, bytes to read=4, error in (no error)=w1131) -> (connection ID out=w1139:refnum<k5>, data out=w1142:string, error out=w1138:errorcluster)  [unwired: 2 out]
            n477 = Type Cast(type=0, x=w1142) -> (*(type *) &x=w1140:i32)
            n478 = TCP Read(connection ID=w1139, bytes to read=w1140, error in (no error)=w1138) -> (connection ID out=w1134:refnum<k5>, data out=w1137:string, error out=w1133:errorcluster)  [unwired: 2 out]
            n479 = call "deleteEndString.vi"("chars to delete"=5, "string in"=w1137) -> ("substring out"=w1136:string)  [unwired: 9 out]
            n480 = local read "Indicators formated"() -> (w1126:cluster{"name":string, "type desc":i16[]}[])
            n481 = call "searchElement.vi"("input"=w1126, "name"=w1136) -> ("output"=w1144:cluster{"name":string, "type desc":i16[]})  [unwired: 9 out]
            n482 = local read "vi reference"() -> (w1125:refnum<vi>)
            n483 = Unbundle By Name(w1144) -> ("name"=w1143:string)
            n484 = invoke class="VI" method="Ctrl Val.Get (Deprecated)"(reference=w1125, "Control Name"=w1143) -> (error out=w1124:errorcluster, "Get Control Value"=w1127:string)  [unwired: 3 in, 3 out]
            n485 = TCP Write(connection ID=w1134, data in=w1127, error in (no error)=w1133) -> (connection ID out=w1129:refnum<k5>, error out=w1130:errorcluster)  [unwired: 2 out]
            n486 = call "setError.vi"("error"=w1124) -> ()  [unwired: 1 out]
          }
          frame "getStringArray2D" {
            n487 = TCP Read(connection ID=w1150, bytes to read=4, error in (no error)=w1149) -> (connection ID out=w1161:refnum<k5>, data out=w1164:string, error out=w1160:errorcluster)  [unwired: 2 out]
            n488 = Type Cast(type=0, x=w1164) -> (*(type *) &x=w1162:i32)
            n489 = TCP Read(connection ID=w1161, bytes to read=w1162, error in (no error)=w1160) -> (connection ID out=w1156:refnum<k5>, data out=w1159:string, error out=w1155:errorcluster)  [unwired: 2 out]
            n490 = local read "Indicators formated"() -> (w1147:cluster{"name":string, "type desc":i16[]}[])
            n491 = call "deleteEndString.vi"("chars to delete"=5, "string in"=w1159) -> ("substring out"=w1158:string)  [unwired: 9 out]
            n492 = call "searchElement.vi"("input"=w1147, "name"=w1158) -> ("output"=w1166:cluster{"name":string, "type desc":i16[]})  [unwired: 9 out]
            n493 = local read "vi reference"() -> (w1148:refnum<vi>)
            n494 = Unbundle By Name(w1166) -> ("name"=w1165:string)
            n495 = invoke class="VI" method="Ctrl Val.Get (Deprecated)"(reference=w1148, "Control Name"=w1165) -> (error out=w1146:errorcluster, "Get Control Value"=w1154:string)  [unwired: 3 in, 3 out]
            n496 = TCP Write(connection ID=w1156, data in=w1154, error in (no error)=w1155) -> (connection ID out=w1153:refnum<k5>, error out=w1152:errorcluster)  [unwired: 2 out]
            n497 = call "setError.vi"("error"=w1146) -> ()  [unwired: 1 out]
          }
          frame "getFloatArray2D" {
            n498 = TCP Read(connection ID=w1173, bytes to read=4, error in (no error)=w1172) -> (connection ID out=w1183:refnum<k5>, data out=w1186:string, error out=w1182:errorcluster)  [unwired: 2 out]
            n499 = Type Cast(type=0, x=w1186) -> (*(type *) &x=w1184:i32)
            n500 = local read "Controls formated"() -> (w1174:cluster{"name":string, "type desc":i16[]}[])
            n501 = TCP Read(connection ID=w1183, bytes to read=w1184, error in (no error)=w1182) -> (connection ID out=w1178:refnum<k5>, data out=w1181:string, error out=w1177:errorcluster)  [unwired: 2 out]
            n502 = call "deleteEndString.vi"("chars to delete"=5, "string in"=w1181) -> ("substring out"=w1180:string)  [unwired: 9 out]
            n503 = local read "vi reference"() -> (w1175:refnum<vi>)
            n504 = call "searchElement.vi"("input"=w1174, "name"=w1180) -> ("output"=w1188:cluster{"name":string, "type desc":i16[]})  [unwired: 9 out]
            n505 = Unbundle By Name(w1188) -> ("name"=w1187:string)
            n506 = invoke class="VI" method="Ctrl Val.Get (Deprecated)"(reference=w1175, "Control Name"=w1187) -> (error out=w1168:errorcluster, "Get Control Value"=w1176:string)  [unwired: 3 in, 3 out]
            n507 = TCP Write(connection ID=w1178, data in=w1176, error in (no error)=w1177) -> (connection ID out=w1170:refnum<k5>, error out=w1171:errorcluster)  [unwired: 2 out]
            n508 = call "setError.vi"("error"=w1168) -> ()  [unwired: 1 out]
          }
        }
        n509 = call "error6662.vi"("input error"=w24) -> ("result"=w21:bool, "output error"=w23:errorcluster)  [unwired: 3 out]
        n510 = call "stopVILV2G.vi"("Mode"=enum16{"Init", "Get", "Set"}."Get") -> ("Stop OUT"=w18:bool)  [unwired: 1 in, 9 out]
        n511 = Compound Arithmetic op=OR(w21, w20, w18) -> (w22:bool)
      }
      n512 = TCP Close Connection(connection ID=w11, error in (no error)=w12) -> (error out=w10:errorcluster)  [unwired: 2 out]
      n513 = call "setError.vi"("error"=w10) -> ()  [unwired: 1 out]
    }
    frame #1 {
      w1191 = u16 1 items=["connectedMsg", "disconnectedMsg", "openVIRefMsg", "closeVIRefMsg"] ("Type of Message")
      n514 = call "setConnectionReport.vi"("string"=w1190, "Type of Message"=w1191) -> ()  [unwired: 10 in]
      n515 = local read "vi reference"() -> (w1200:refnum<vi>)
      n516 = property class="VI"(reference=w1200) -> (reference out=w1199:refnum<vi>, error out=w1198:errorcluster, "Front Panel.Open"=w1201:bool)  [unwired: 1 in]
      n517 = case shown="True" w1201 {
        tunnel: w1199 -> [w1203 w1207]
        tunnel: w1198 -> [w1202 w1204]
        tunnel: [w1203 w1206] -> w1197
        tunnel: [w1202 w1205] -> w1196
        frame False {
        }
        frame True {
          n518 = invoke class="VI" method="FP.Close"(reference=w1207, error in=w1204) -> (reference out=w1206:refnum<vi>, error out=w1205:errorcluster)  [unwired: 1 in, 1 out]
        }
      }
      n519 = property class="VI"(reference=w1197, error in=w1196) -> (reference out=w1195:refnum<vi>, error out=w1194:errorcluster, "Exec.State"=w1193:T3)
      n520 = local write "Execution: State VI"(w1193) -> ()
      n521 = Close Reference(reference=w1195, error in (no error)=w1194) -> (error out=w1192:errorcluster)
      n522 = call "setError.vi"("error"=w1192) -> ()  [unwired: 1 out]
    }
  }
